vi "Strategy 5_Autotuning PID_With GUI - Copy (2).vi"() -> ()   [LabVIEW 2018]
doc: "This example demonstrates how to use the PID Design function to obtain PID parameters based on measured process."
uses:
  <vilib>/DAQmx/write.llb/DAQmx Write (Digital 1D Bool 1Chan 1Samp).vi
  <vilib>/Instr/_visa.llb/VISA Configure Serial Port (Instr).vi
  <vilib>/DAQmx/create/channels.llb/DAQmx Create Channel (DO-Digital Output).vi
  <vilib>/DAQmx/miscellaneous.llb/DAQmx Fill In Error Info.vi
  <vilib>/addons/control/pid/pid.llb/PID Advanced (DBL).vi
  <vilib>/addons/control/pid/autopid.llb/PID Autotuning Design (Ziegler-Nichols).vi
  <vilib>/addons/control/pid/autopid.llb/PID Autotuning Design (Cohen-Coon).vi
  <vilib>/addons/control/pid/autopid.llb/PID Autotuning Design (Chien-Hrones-Reswick).vi
  <vilib>/addons/control/pid/autopid.llb/PID Autotuning Design (Internal Model Control).vi
  <vilib>/addons/control/pid/NI_PID_autopid.lvlib
  <vilib>/addons/control/pid/NI_PID_pid.lvlib
  <vilib>/ptbypt/NI_PtbyPt.lvlib
panel:
  out "?":bool
  in  "Muscle Control":T1(tab)=enum."M-11"
  out "Tuned PID gains 8":T2={"proportional gain (Kc)"=1.9838195929127882, "integral time (Ti, min)"=0.01995856284686879, "derivative time (Td, min)"=0.0} {"derivative time (Td, min)" format="%#.6g"; "integral time (Ti, min)" format="%#.6g"; "proportional gain (Kc)" format="%#.6g"}
  in  "Accept gain 8":bool
  in  "Control 8":T3(tab)
  in  "Ziegler-Nichols speed 8":u16(ring) items=["Fast", "Normal", "Slow"]
  in  "Tuning specifications 8":u16(ring) items=["Regulator - 0 %", "Regulator -  20%", "Servo - 0%", "Servo - 20%"]
  in  "Multiplicative factor 8":dbl(slide)=1.0 scale=0.01..100.0
  in  "Type of controller 8":u16(ring)=2 items=["P", "PI", "PID"]
  in  "Stop 8":bool
  in  "PID Gains 8":T2={"proportional gain (Kc)"=0.1625, "integral time (Ti, min)"=1.25, "derivative time (Td, min)"=0.0} {"derivative time (Td, min)" format="%#.6g"; "integral time (Ti, min)" format="%#.6g"; "proportional gain (Kc)" format="%#.6g"}
  in  "Autotune 8":bool
  in  "Reinitialize 8":bool
  in  "Excitation 8":dbl=0.5 format="%.2f"
  in  "Automatic 8":bool=TRUE
  in  "MV: 8":dbl(slide)=20.39115328927357 scale=-100.0..100.0
  in  "Set Point 8":dbl(slide) scale=0.0..30.0
  out "PWM Output 8":bool
  out "Real time Data 8":dbl[][](graph)
  in  "Median sample length 17":i32=100
  in  "INLET 2 ON/OFF 2":bool=TRUE
  out "Tuned PID gains 7":T2={"proportional gain (Kc)"=1.9838195929127882, "integral time (Ti, min)"=0.01995856284686879, "derivative time (Td, min)"=0.0} {"derivative time (Td, min)" format="%#.6g"; "integral time (Ti, min)" format="%#.6g"; "proportional gain (Kc)" format="%#.6g"}
  in  "Accept gain 7":bool
  in  "Control 7":T3(tab)
  in  "Ziegler-Nichols speed 7":u16(ring) items=["Fast", "Normal", "Slow"]
  in  "Tuning specifications 7":u16(ring) items=["Regulator - 0 %", "Regulator -  20%", "Servo - 0%", "Servo - 20%"]
  in  "Multiplicative factor 7":dbl(slide)=1.0 scale=0.01..100.0
  in  "Type of controller 7":u16(ring)=2 items=["P", "PI", "PID"]
  in  "Stop 7":bool
  in  "PID Gains 7":T2={"proportional gain (Kc)"=0.1625, "integral time (Ti, min)"=1.25, "derivative time (Td, min)"=0.0} {"derivative time (Td, min)" format="%#.6g"; "integral time (Ti, min)" format="%#.6g"; "proportional gain (Kc)" format="%#.6g"}
  in  "Autotune 7":bool
  in  "Reinitialize 7":bool
  in  "Excitation 7":dbl=0.5 format="%.2f"
  in  "Automatic 7":bool=TRUE
  in  "MV: 7":dbl(slide)=20.39115328927357 scale=-100.0..100.0
  in  "Set Point 7":dbl(slide) scale=0.0..30.0
  out "PWM Output 7":bool
  out "Real time Data 7":dbl[][](graph)
  in  "Median sample length 16":i32=100
  in  "INLET 7 ON/OFF 2":bool=TRUE
  out "Tuned PID gains 6":T2={"proportional gain (Kc)"=1.9838195929127882, "integral time (Ti, min)"=0.01995856284686879, "derivative time (Td, min)"=0.0} {"derivative time (Td, min)" format="%#.6g"; "integral time (Ti, min)" format="%#.6g"; "proportional gain (Kc)" format="%#.6g"}
  in  "Accept gain 6":bool
  in  "Control 6":T3(tab)
  in  "Ziegler-Nichols speed 6":u16(ring) items=["Fast", "Normal", "Slow"]
  in  "Tuning specifications 6":u16(ring) items=["Regulator - 0 %", "Regulator -  20%", "Servo - 0%", "Servo - 20%"]
  in  "Multiplicative factor 6":dbl(slide)=1.0 scale=0.01..100.0
  in  "Type of controller 6":u16(ring)=2 items=["P", "PI", "PID"]
  in  "Stop 6":bool
  in  "PID Gains 6":T2={"proportional gain (Kc)"=0.1625, "integral time (Ti, min)"=1.25, "derivative time (Td, min)"=0.0} {"derivative time (Td, min)" format="%#.6g"; "integral time (Ti, min)" format="%#.6g"; "proportional gain (Kc)" format="%#.6g"}
  in  "Autotune 6":bool
  in  "Reinitialize 6":bool
  in  "Excitation 6":dbl=0.5 format="%.2f"
  in  "Automatic 6":bool=TRUE
  in  "MV: 6":dbl(slide)=20.39115328927357 scale=-100.0..100.0
  in  "Set Point 6":dbl(slide) scale=0.0..30.0
  out "PWM Output 6":bool
  out "Real time Data 6":dbl[][](graph)
  in  "Median sample length 15":i32=100
  in  "INLET 6 ON/OFF 2":bool=TRUE
  out "Tuned PID gains 5":T2={"proportional gain (Kc)"=1.9838195929127882, "integral time (Ti, min)"=0.01995856284686879, "derivative time (Td, min)"=0.0} {"derivative time (Td, min)" format="%#.6g"; "integral time (Ti, min)" format="%#.6g"; "proportional gain (Kc)" format="%#.6g"}
  in  "Accept gain 5":bool
  in  "Control 5":T3(tab)
  in  "Ziegler-Nichols speed 5":u16(ring) items=["Fast", "Normal", "Slow"]
  in  "Tuning specifications 5":u16(ring) items=["Regulator - 0 %", "Regulator -  20%", "Servo - 0%", "Servo - 20%"]
  in  "Multiplicative factor 5":dbl(slide)=1.0 scale=0.01..100.0
  in  "Type of controller 5":u16(ring)=2 items=["P", "PI", "PID"]
  in  "Stop 5":bool
  in  "PID Gains 5":T2={"proportional gain (Kc)"=0.1625, "integral time (Ti, min)"=1.25, "derivative time (Td, min)"=0.0} {"derivative time (Td, min)" format="%#.6g"; "integral time (Ti, min)" format="%#.6g"; "proportional gain (Kc)" format="%#.6g"}
  in  "Autotune 5":bool
  in  "Reinitialize 5":bool
  in  "Excitation 5":dbl=0.5 format="%.2f"
  in  "Automatic 5":bool=TRUE
  in  "MV: 5":dbl(slide)=20.39115328927357 scale=-100.0..100.0
  in  "Set Point 5":dbl(slide) scale=0.0..30.0
  out "PWM Output 5":bool
  out "Real time Data 5":dbl[][](graph)
  in  "Median sample length 14":i32=100
  in  "INLET 8 ON/OFF 2":bool=TRUE
  out "Tuned PID gains 4":T2={"proportional gain (Kc)"=1.9838195929127882, "integral time (Ti, min)"=0.01995856284686879, "derivative time (Td, min)"=0.0} {"derivative time (Td, min)" format="%#.6g"; "integral time (Ti, min)" format="%#.6g"; "proportional gain (Kc)" format="%#.6g"}
  in  "Accept gain 4":bool
  in  "Control 4":T3(tab)
  in  "Ziegler-Nichols speed 4":u16(ring) items=["Fast", "Normal", "Slow"]
  in  "Tuning specifications 4":u16(ring) items=["Regulator - 0 %", "Regulator -  20%", "Servo - 0%", "Servo - 20%"]
  in  "Multiplicative factor 4":dbl(slide)=1.0 scale=0.01..100.0
  in  "Type of controller 4":u16(ring)=2 items=["P", "PI", "PID"]
  in  "Stop 4":bool
  in  "PID Gains 4":T2={"proportional gain (Kc)"=0.1625, "integral time (Ti, min)"=1.25, "derivative time (Td, min)"=0.0} {"derivative time (Td, min)" format="%#.6g"; "integral time (Ti, min)" format="%#.6g"; "proportional gain (Kc)" format="%#.6g"}
  in  "Autotune 4":bool
  in  "Reinitialize 4":bool
  in  "Excitation 4":dbl=0.5 format="%.2f"
  in  "Automatic 4":bool=TRUE
  in  "MV: 4":dbl(slide)=20.39115328927357 scale=-100.0..100.0
  in  "Set Point 4":dbl(slide) scale=0.0..30.0
  out "PWM Output 4":bool
  out "Real time Data 4":dbl[][](graph)
  in  "Median sample length 9":i32=100
  in  "INLET 9 ON/OFF 2":bool=TRUE
  out "Tuned PID gains 3":T2={"proportional gain (Kc)"=1.9838195929127882, "integral time (Ti, min)"=0.01995856284686879, "derivative time (Td, min)"=0.0} {"derivative time (Td, min)" format="%#.6g"; "integral time (Ti, min)" format="%#.6g"; "proportional gain (Kc)" format="%#.6g"}
  in  "Accept gain 3":bool
  in  "Control 3":T3(tab)
  in  "Ziegler-Nichols speed 3":u16(ring) items=["Fast", "Normal", "Slow"]
  in  "Tuning specifications 3":u16(ring) items=["Regulator - 0 %", "Regulator -  20%", "Servo - 0%", "Servo - 20%"]
  in  "Multiplicative factor 3":dbl(slide)=1.0 scale=0.01..100.0
  in  "Type of controller 3":u16(ring)=2 items=["P", "PI", "PID"]
  in  "Stop 3":bool
  in  "PID Gains 3":T2={"proportional gain (Kc)"=0.1625, "integral time (Ti, min)"=1.25, "derivative time (Td, min)"=0.0} {"derivative time (Td, min)" format="%#.6g"; "integral time (Ti, min)" format="%#.6g"; "proportional gain (Kc)" format="%#.6g"}
  in  "Autotune 3":bool
  in  "Reinitialize 3":bool
  in  "Excitation 3":dbl=0.5 format="%.2f"
  in  "Automatic 3":bool=TRUE
  in  "MV: 3":dbl(slide)=20.39115328927357 scale=-100.0..100.0
  in  "Set Point 3":dbl(slide) scale=0.0..30.0
  out "PWM Output 3":bool
  out "Real time Data 3":dbl[][](graph)
  in  "Median sample length 13":i32=100
  in  "INLET 10 ON/OFF":bool=TRUE
  in  "INLET":bool=TRUE
  out "PWM Output":bool
  out "Real time Data":dbl[][](graph)
  in  "MV:":dbl(slide)=20.39115328927357 scale=-100.0..100.0
  in  "Set Point":dbl(slide) scale=0.0..30.0
  in  "Median sample length":i32=100
  in  "Excitation":dbl=0.5 format="%.2f"
  in  "Type of controller":u16(ring)=2 items=["P", "PI", "PID"]
  in  "Control":T3(tab)
  in  "Ziegler-Nichols speed":u16(ring) items=["Fast", "Normal", "Slow"]
  in  "Tuning specifications":u16(ring) items=["Regulator - 0 %", "Regulator -  20%", "Servo - 0%", "Servo - 20%"]
  in  "Multiplicative factor":dbl(slide)=1.0 scale=0.01..100.0
  in  "Automatic":bool=TRUE
  in  "Reinitialize":bool
  in  "Accept gain":bool
  out "Tuned PID gains":T2={"proportional gain (Kc)"=1.9838195929127882, "integral time (Ti, min)"=0.01995856284686879, "derivative time (Td, min)"=0.0} {"derivative time (Td, min)" format="%#.6g"; "integral time (Ti, min)" format="%#.6g"; "proportional gain (Kc)" format="%#.6g"}
  in  "Autotune":bool
  in  "PID Gains":T2={"proportional gain (Kc)"=0.1625, "integral time (Ti, min)"=1.25, "derivative time (Td, min)"=0.0} {"derivative time (Td, min)" format="%#.6g"; "integral time (Ti, min)" format="%#.6g"; "proportional gain (Kc)" format="%#.6g"}
  in  "Stop":bool
  out "Tuned PID gains 2":T2={"proportional gain (Kc)"=1.9838195929127882, "integral time (Ti, min)"=0.01995856284686879, "derivative time (Td, min)"=0.0} {"derivative time (Td, min)" format="%#.6g"; "integral time (Ti, min)" format="%#.6g"; "proportional gain (Kc)" format="%#.6g"}
  in  "Accept gain 2":bool
  in  "Control 2":T3(tab)
  in  "Ziegler-Nichols speed 2":u16(ring) items=["Fast", "Normal", "Slow"]
  in  "Tuning specifications 2":u16(ring) items=["Regulator - 0 %", "Regulator -  20%", "Servo - 0%", "Servo - 20%"]
  in  "Multiplicative factor 2":dbl(slide)=1.0 scale=0.01..100.0
  in  "Type of controller 2":u16(ring)=2 items=["P", "PI", "PID"]
  in  "Stop 2":bool
  in  "PID Gains 2":T2={"proportional gain (Kc)"=0.1625, "integral time (Ti, min)"=1.25, "derivative time (Td, min)"=0.0} {"derivative time (Td, min)" format="%#.6g"; "integral time (Ti, min)" format="%#.6g"; "proportional gain (Kc)" format="%#.6g"}
  in  "Autotune 2":bool
  in  "Reinitialize 2":bool
  in  "Excitation 2":dbl=0.5 format="%.2f"
  in  "Automatic 2":bool=TRUE
  in  "MV: 2":dbl(slide)=20.39115328927357 scale=-100.0..100.0
  in  "Set Point 2":dbl(slide) scale=0.0..30.0
  out "PWM Output 2":bool
  out "Real time Data 2":dbl[][](graph)
  in  "Median sample length 12":i32=100
  in  "INLET 12 ON/OFF":bool=TRUE
  in  "M-11":i32=5
  in  "M-12":i32=5
  in  "M-10":i32=5
  in  "M-9":i32=5
  in  "M-8":i32=5
  in  "M-6":i32=5
  in  "M-7":i32=5
  in  "M-2":i32=5
  out "Identified Plant Parameters":T4={"Plant Gain (K)"=1.7609511324977591, "Time Constant (T)"=1.9621978490901302, "Dead Time (L)"=0.22467425343567116}
  out "Control Output":dbl[](graph)
  out "Measurement":dbl[](graph)
  out "Stimulus operating point":dbl=20.314221540357543
  out "Response operating point":dbl=51.08345461694337
  out "Stimulus operating point 2":dbl=20.314221540357543
  out "Response operating point 2":dbl=51.08345461694337
  out "Identified Plant Parameters 2":T4={"Plant Gain (K)"=1.7609511324977591, "Time Constant (T)"=1.9621978490901302, "Dead Time (L)"=0.22467425343567116}
  out "Control Output 2":dbl[](graph)
  out "Measurement 2":dbl[](graph)
  out "Stimulus operating point 3":dbl=20.314221540357543
  out "Response operating point 3":dbl=51.08345461694337
  out "Identified Plant Parameters 3":T4={"Plant Gain (K)"=1.7609511324977591, "Time Constant (T)"=1.9621978490901302, "Dead Time (L)"=0.22467425343567116}
  out "Control Output 3":dbl[](graph)
  out "Measurement 3":dbl[](graph)
  out "Stimulus operating point 4":dbl=20.314221540357543
  out "Response operating point 4":dbl=51.08345461694337
  out "Identified Plant Parameters 4":T4={"Plant Gain (K)"=1.7609511324977591, "Time Constant (T)"=1.9621978490901302, "Dead Time (L)"=0.22467425343567116}
  out "Control Output 4":dbl[](graph)
  out "Measurement 4":dbl[](graph)
  out "Stimulus operating point 5":dbl=20.314221540357543
  out "Response operating point 5":dbl=51.08345461694337
  out "Identified Plant Parameters 5":T4={"Plant Gain (K)"=1.7609511324977591, "Time Constant (T)"=1.9621978490901302, "Dead Time (L)"=0.22467425343567116}
  out "Control Output 5":dbl[](graph)
  out "Measurement 5":dbl[](graph)
  out "Stimulus operating point 6":dbl=20.314221540357543
  out "Response operating point 6":dbl=51.08345461694337
  out "Identified Plant Parameters 6":T4={"Plant Gain (K)"=1.7609511324977591, "Time Constant (T)"=1.9621978490901302, "Dead Time (L)"=0.22467425343567116}
  out "Control Output 6":dbl[](graph)
  out "Measurement 6":dbl[](graph)
  out "Stimulus operating point 7":dbl=20.314221540357543
  out "Response operating point 7":dbl=51.08345461694337
  out "Identified Plant Parameters 7":T4={"Plant Gain (K)"=1.7609511324977591, "Time Constant (T)"=1.9621978490901302, "Dead Time (L)"=0.22467425343567116}
  out "Control Output 7":dbl[](graph)
  out "Measurement 7":dbl[](graph)
  out "Stimulus operating point 8":dbl=20.314221540357543
  out "Response operating point 8":dbl=51.08345461694337
  out "Identified Plant Parameters 8":T4={"Plant Gain (K)"=1.7609511324977591, "Time Constant (T)"=1.9621978490901302, "Dead Time (L)"=0.22467425343567116}
  out "Control Output 8":dbl[](graph)
  out "Measurement 8":dbl[](graph)
  in  "XYZAER":T5(array[cluster]) {"r" format="%1_6f"; "e" format="%1_6f"; "a" format="%1_6f"; "z" format="%1_6f"; "y" format="%1_6f"; "x" format="%1_6f"}
  out "Connected":bool
  out "Start Time Text":string
  out "Stop Time Text":string
  out "Elapsed Time Text":string
  out "HostFrameCount":u32
  out "Running":bool
  out "Loop Iter":i32
  out "PnoData":bool
  in  "stop":bool
  out "error out":errorcluster {"code" format="%.0x"}
  out "Position Sensor Data":cluster{dbl, "x":sgl}[](graph)
  out "Sensor Raw Value 2":i32
  in  "COM Port-Sensor 2":refnum<visa-resource-name>="COM5"
  in  "upper/lower infle":enum32{"Page 1", "Page 2"}(tab)
  out "Force in Kilograms":dbl(graph)
  out "Force in Newtons":dbl(graph)
  in  "lower/upper infle":enum32{"Page 1", "Page 2"}(tab)
  out "Force in Newtons 2":dbl(graph)
  out "Force in Kilograms 2":dbl(graph)
  in  "COM Port-Sensor 1":refnum<visa-resource-name>="COM4"
  out "Sensor Raw Value":i32
  in  "Tab Control":T6(tab)
  in  "Instructions":string="Overview: This example demonstrates how to use the PID Autotuning Design to obtain PID parameters based on setpoint and process variable collected in another loop.\nInstructions:\n1. Run the VI and wait until the process variable (PV) reaches near setpoint (SP).\n2.  In the PID Autotuning Design section, select the type of algorithm, type of controller and excitation amplitude for the 'open loop step response'. Then, click Autotune to start the process. Select the Identified Plant Parameter tab and see the results from the identification.\n3.  When the tuned PID gains do not change anymore, the identification is done and you have the option to accept by clicking Accept gain, which will transfer the new gain to PID Gains.\n4. Click the Autotune button again to go back to the automatic control state. You can try different options and repeat this process.\n5. Click Stop to stop the VI.\n"
  in  "Instructions 2":string="Overview: This example demonstrates how to use the PID Autotuning Design to obtain PID parameters based on setpoint and process variable collected in another loop.\nInstructions:\n1. Run the VI and wait until the process variable (PV) reaches near setpoint (SP).\n2.  In the PID Autotuning Design section, select the type of algorithm, type of controller and excitation amplitude for the 'open loop step response'. Then, click Autotune to start the process. Select the Identified Plant Parameter tab and see the results from the identification.\n3.  When the tuned PID gains do not change anymore, the identification is done and you have the option to accept by clicking Accept gain, which will transfer the new gain to PID Gains.\n4. Click the Autotune button again to go back to the automatic control state. You can try different options and repeat this process.\n5. Click Stop to stop the VI.\n"
  in  "Instructions 3":string="Overview: This example demonstrates how to use the PID Autotuning Design to obtain PID parameters based on setpoint and process variable collected in another loop.\nInstructions:\n1. Run the VI and wait until the process variable (PV) reaches near setpoint (SP).\n2.  In the PID Autotuning Design section, select the type of algorithm, type of controller and excitation amplitude for the 'open loop step response'. Then, click Autotune to start the process. Select the Identified Plant Parameter tab and see the results from the identification.\n3.  When the tuned PID gains do not change anymore, the identification is done and you have the option to accept by clicking Accept gain, which will transfer the new gain to PID Gains.\n4. Click the Autotune button again to go back to the automatic control state. You can try different options and repeat this process.\n5. Click Stop to stop the VI.\n"
  # "Pressure Alarm"
  # "Position Sensor Data"
  # "Force Sensor Data"
  # "PID Controller"
  # "PID Autotuning Design"
  # "No additional parameters"
  # "PID Controller"
  # "PID Autotuning Design"
  # "No additional parameters"
  # "PID Controller"
  # "PID Autotuning Design"
  # "No additional parameters"
  # "Muscle Control"
  # "PID Controller"
  # "PID Autotuning Design"
  # "No additional parameters"
  # "PID Controller"
  # "PID Autotuning Design"
  # "No additional parameters"
  # "PID Controller"
  # "PID Autotuning Design"
  # "No additional parameters"
  # "Muscle Control"
  # "PID Controller"
  # "PID Autotuning Design"
  # "No additional parameters"
  # "PID Controller"
  # "PID Autotuning Design"
  # "No additional parameters"
  # "Pressure Cut Off to trigger the alarm"
  # "M-11"
  # "M-12"
  # "M-10"
  # "M-9"
  # "M-8"
  # "M-6"
  # "M-7"
  # "M-2"
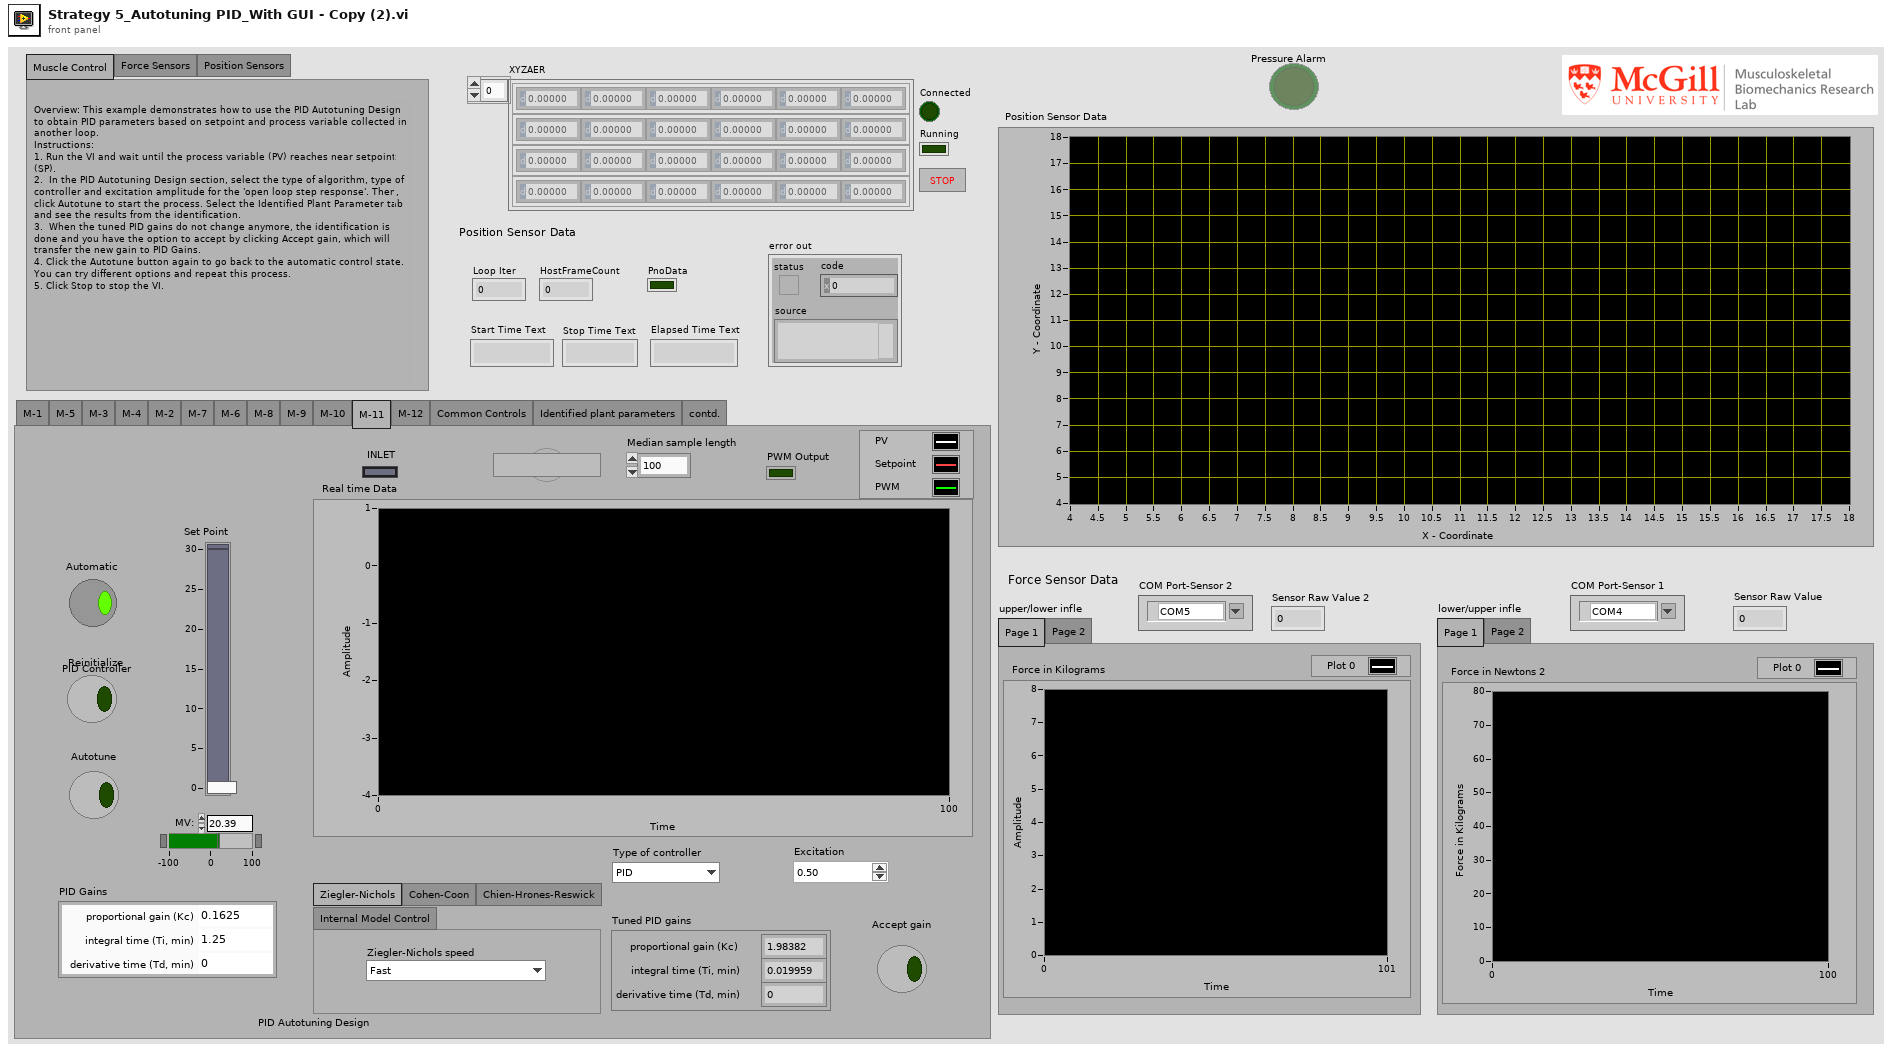
[diagram p1: front panel]
types:
  T1 = enum32{"M-1", "M-5", "M-3", "M-4", "M-2", "M-7", "M-6", "M-8", "M-9", "M-10", "M-11", "M-12", "Common Controls", "Identified plant parameters", "contd."}
  T2 = cluster{"proportional gain (Kc)":dbl, "integral time (Ti, min)":dbl, "derivative time (Td, min)":dbl}
  T3 = enum32{"Ziegler-Nichols", "Cohen-Coon", "Chien-Hrones-Reswick", "Internal Model Control"}
  T4 = cluster{"Plant Gain (K)":dbl, "Time Constant (T)":dbl, "Dead Time (L)":dbl}
  T5 = cluster{"x":sgl, "y":sgl, "z":sgl, "a":sgl, "e":sgl, "r":sgl}[]
  T6 = enum32{"Muscle Control", "Force Sensors", "Position Sensors"}
  T7 = cluster{"static gain":dbl, "lag (s)":dbl, "deadtime (s)":dbl, "load":dbl, "deadband":dbl, "sensor noise":dbl, "initial PV":dbl, "plant noise":dbl}
  T8 = cluster{"x":sgl, "y":sgl, "z":sgl, "a":sgl, "e":sgl, "r":sgl}
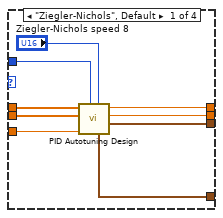
[diagram p2: hidden frame]
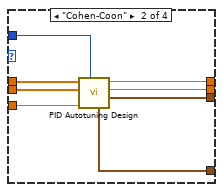
[diagram p3: hidden frame]
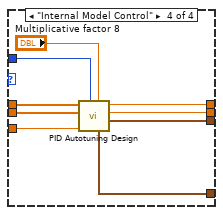
[diagram p4: hidden frame]
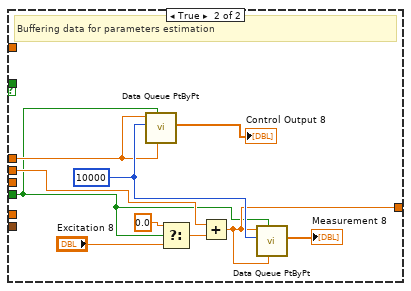
[diagram p6: hidden frame]
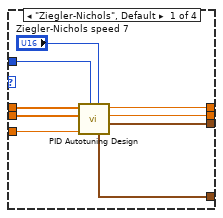
[diagram p7: hidden frame]
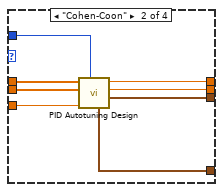
[diagram p8: hidden frame]
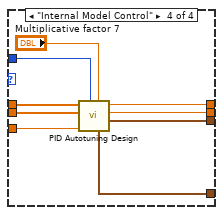
[diagram p9: hidden frame]
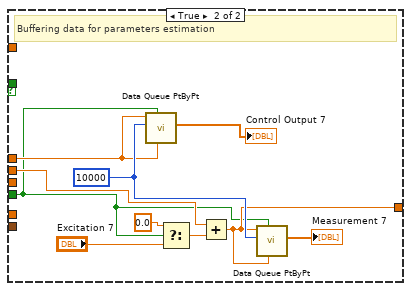
[diagram p11: hidden frame]
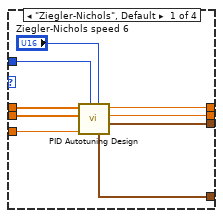
[diagram p12: hidden frame]
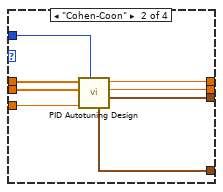
[diagram p13: hidden frame]
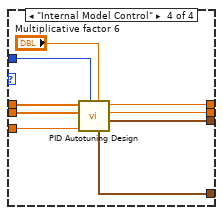
[diagram p14: hidden frame]
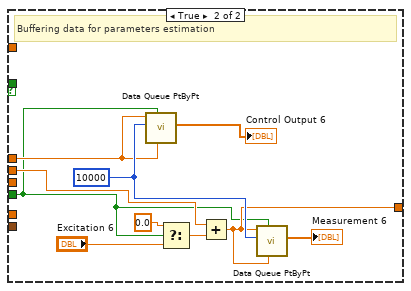
[diagram p16: hidden frame]
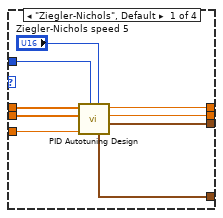
[diagram p17: hidden frame]
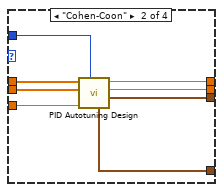
[diagram p18: hidden frame]
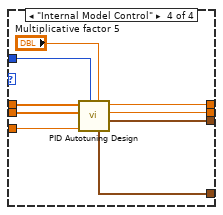
[diagram p19: hidden frame]
diagram:
  w3 = 0.0 ("output")
  w6 = FALSE ("Stop")
  w9 = 0.0 ("output")
  w12 = FALSE ("Stop")
  w15 = 0.0 ("output")
  w18 = FALSE ("Stop")
  w21 = 0.0 ("output")
  w24 = FALSE ("Stop")
  w27 = 0.0 ("output")
  w30 = FALSE ("Stop")
  w33 = 0.0 ("output")
  w36 = FALSE ("Stop")
  w39 = 0.0 ("output")
  w42 = FALSE ("Stop")
  w50 = 2400  # BufferFrameCount
  w84 = 0.0 ("output")
  w87 = FALSE ("Stop")
  # "Muscle-2 PID CONTROL LOOP (Auto Tuning)"
  # "Muscle-7 PID CONTROL LOOP (Auto Tuning)"
  # "Muscle-6 PID CONTROL LOOP (Auto Tuning)"
  # "Muscle-8 PID CONTROL LOOP (Auto Tuning)"
  # "Muscle-9 PID CONTROL LOOP (Auto Tuning)"
  # "Muscle-10 PID CONTROL LOOP (Auto Tuning)"
  # "Muscle-12 PID CONTROL LOOP (Auto Tuning)"
  # "Muscle-11 PID CONTROL LOOP (Auto Tuning)"
  # "FORCE SENSOR CONTROL LOOP"
  # "POSITION SENSOR CONTROL LOOP"
  # "Pressure Alarm"
  # "8. Close Tracker connection."
  # "3. Query Max num sensors supported by the tracker."
  # "4. Allocate raw buffer to hold 2400 frames of data."
  # "5. Start Continuous mode."
  # "7. Stop Continuous mode."
  # "6. Start the loop. Loop exits when Stop Button is hit."
  n1 = call "DAQ Assistant"() -> ("data"=w1:dynamicdata)  [unwired: 17 in, 2 out]
  n2 = while {
    shift-left: 0.0 ("Plant Output") -> [w153]
    shift-right: [w148] -> _
    tunnel: w18 -> [_]
    shift-right: [w134] -> _
    shift-left: 0.01 -> [w132]
    shift-right: [w106] -> _
    shift-left: TRUE -> [w131]
    shift-right: [w108] -> _
    shift-left: w15 -> [w130]
    shift-right: [w133] -> _
    shift-left: w15 -> [w129]
    tunnel: [w103] -> w14
    tunnel: w1 -> [w89]
    stop <- "Stop 6" stop-if-true
    w94 = 1 items=["one channel for each line", "one channel for all lines"] ("line grouping")
    w103 = 0.05 ("Sampling Time dt (s)")
    w112 = 1 items=["one channel for each line", "one channel for all lines"] ("line grouping")
    w120 = 0.5 ("x")
    w147 = T7 {"static gain"=2.5, "lag (s)"=2.5, "deadtime (s)"=0.01, "load"=0.0, "deadband"=0.0, "sensor noise"=0.0, "initial PV"=30.0, "plant noise"=0.0}  # Process parameters
    w149 = FALSE  # Integrator ?
    # "C."
    # "Inlet 11"
    # "Exhaust 6"
    # "B."
    # "A."
    # "A.Output to PWM Logic \nB. Simulated Plant\nC. Draw Chart"
    # "Main PID Loop Control"
    n3 = Multiply(x=w103, y=1000.0) -> (x*y=w146:dbl)
    n4 = Not(x="Autotune 6") -> (.not. x?=w150:bool)
    n5 = feedback #1() -> (w155:bool)  [unwired: 1 in]
    n6 = feedback-in #1("Autotune 6") -> ()
    n7 = Wait Until Next ms Multiple(millisecond multiple=w146) -> ()  [unwired: 1 out]
    n8 = Exclusive Or(1:w155, 2:"Autotune 6") -> (0:w154:bool)
    n9 = feedback #2() -> (w152:dbl)  [unwired: 1 in]
    n10 = Multiply(x=w89, y=-1000.0) -> (x*y=w136:dynamicdata)
    n11 = call <vilib>:"Median PtByPt.vi"("sample length"="Median sample length 15", "x"=w136) -> ("median"=w135:dbl)  [unwired: 2 in, 1 out]
    n12 = Square(x=w135) -> (x^2=w143:dbl)
    n13 = Multiply(x=w135, y=-39.646) -> (x*y=w139:dbl)
    n14 = Multiply(x=w143, y=0.2324) -> (x*y=w140:dbl)
    n15 = Add(x=w139, y=w140) -> (x+y=w138:dbl)
    n16 = Add(x=1678.0, y=w138) -> (x+y=w101:dbl)
    n17 = case shown="False" "Autotune 6" {
      tunnel: w103 -> [w170 _]
      tunnel: [w159 w175] -> w108
      tunnel: w153 -> [_ w174]
      tunnel: "PID Gains 6" -> [w169 _]
      tunnel: "Reinitialize 6" -> [w166 _]
      tunnel: w154 -> [w168 w173]
      tunnel: w152 -> [_ w177]
      tunnel: w101 -> [w162 _]
      tunnel: "Set Point 6" -> [w161 _]
      frame False {
        # "This code is to have 'bumpless' transfer from autotuning"
        n18 = Not(x=w168) -> (.not. x?=w165:bool)
        n19 = And(x="Automatic 6", y=w165) -> (x .and. y?=w167:bool)
        n20 = call-poly <vilib>:"PID Advanced.vi"("setpoint"=w161, "auto? (T)"=w167, "manual control"="MV: 6", "process variable"=w162, "alpha"=10.0, "PID gains"=w169, "dt (s)"=w170, "reinitialize? (F)"=w166) -> ("output"=w159:dbl)  [unwired: 6 in, 1 out]
      }
      frame True {
        w180 = 10000 ("sample length")
        # "Buffering data for parameters estimation"
        n21 = call <vilib>:"Data Queue PtByPt.vi"("initial queue element"=w174, "initialize"=w173, "sample length"=w180, "input data point"=w174) -> ("Current Queue"=→"Control Output 6":dbl[])  [unwired: 3 in, 4 out]
        n22 = Select(t=0.0, s=w173, f="Excitation 6") -> (s? t:f=w178:dbl)
        n23 = Add(x=w177, y=w178) -> (x+y=w175:dbl)
        n24 = call <vilib>:"Data Queue PtByPt.vi"("initial queue element"=w175, "initialize"=w173, "sample length"=w180, "input data point"=w175) -> ("Current Queue"=→"Measurement 6":dbl[])  [unwired: 3 in, 4 out]
      }
    }
    n25 = feedback-in #2(w108, w150) -> ()
    n26 = Greater?(x=w101, y="M-6") -> ()  [unwired: 1 out]
    n27 = Add(x=w132, y=w120) -> (x+y=w121:dbl)
    n28 = Subtract(x=w132, y=w120) -> (x-y=w119:dbl)
    n29 = Equal?(x=w130, y=w108) -> (x = y?=w127:bool)
    n30 = Greater?(x=w108, y=w130) -> (0:w126:bool)
    n31 = Select(t=w131, s=w127, f=w126) -> (s? t:f=w106:bool)
    "PWM Output 6" <- w106
    n32 = call "Plant System.vi"("Integrator ?"=w149, "Plant Input"=w108, "dt (s)"=w103, "process parameters"=w147) -> ("Plant Output"=w148:dbl)  [unwired: 11 in]
    n33 = Increment(x="Set Point 6") -> (x+1=w125:dbl)
    n34 = Decrement(x="Set Point 6") -> (x-1=w124:dbl)
    n35 = Select(t=w121, s=w106, f=w119) -> (s? t:f=w134:dbl)
    n36 = Select(t=w125, s=w106, f=w124) -> (s? t:f=w123:dbl)
    n37 = Not(x=w106) -> (.not. x?=w105:bool)
    n38 = call-poly <vilib>:"DAQmx Create Virtual Channel.vi"("lines"=tag "cDAQ1Mod1/port0/line4", "line grouping"=w112) -> ("task out"=w114:refnum<k21>, "error out"=w113:errorcluster)  [unwired: 12 in]
    n39 = call-poly <vilib>:"DAQmx Create Virtual Channel.vi"("lines"=tag "cDAQ1Mod2/port0/line4", "line grouping"=w94) -> ("task out"=w96:refnum<k21>, "error out"=w95:errorcluster)  [unwired: 12 in]
    n40 = Build Array(w101, "Set Point 6", w123) -> (w122:dbl[])
    n41 = Initialize Array("INLET 6 ON/OFF 2", 1 ("dimension size")) -> (w91:bool[])
    n42 = Initialize Array(w105, 1 ("dimension size")) -> (w109:bool[])
    n43 = local write "MV: 6"(w108) -> ()
    n44 = Add(x=w129, y=w132) -> (x+y=w133:dbl)
    n45 = Build Array(w122) -> (→"Real time Data 6":dbl[][])
    n46 = call-poly <vilib>:"DAQmx Write.vi"("task/channels in"=w114, "auto start"=TRUE, "data"=w109, "error in"=w113) -> ("task out"=w116:refnum<k21>, "error out"=w117:errorcluster)  [unwired: 9 in, 1 out]
    n47 = call-poly <vilib>:"DAQmx Write.vi"("task/channels in"=w96, "auto start"=TRUE, "data"=w91, "error in"=w95) -> ("task out"=w98:refnum<k21>, "error out"=w99:errorcluster)  [unwired: 9 in, 1 out]
    n48 = call <vilib>:"DAQmx Clear Task.vi"("task in"=w116, "error in"=w117) -> ("error out"=w111:errorcluster)  [unwired: 13 in]
    n49 = call <vilib>:"DAQmx Clear Task.vi"("task in"=w98, "error in"=w99) -> ("error out"=w93:errorcluster)  [unwired: 13 in]
    n50 = call <vilib>:"Simple Error Handler.vi"("error in (no error)"=w111) -> ()  [unwired: 4 in, 5 out]
    n51 = call <vilib>:"Simple Error Handler.vi"("error in (no error)"=w93) -> ()  [unwired: 4 in, 5 out]
  }
  n52 = while {
    shift-left: 0.0 ("Plant Output") -> [w245]
    shift-right: [w240] -> _
    tunnel: w30 -> [_]
    shift-right: [w226] -> _
    shift-left: 0.01 -> [w224]
    shift-right: [w198] -> _
    shift-left: TRUE -> [w223]
    shift-right: [w200] -> _
    shift-left: w27 -> [w222]
    shift-right: [w225] -> _
    shift-left: w27 -> [w221]
    tunnel: [w195] -> w26
    tunnel: w1 -> [w181]
    stop <- "Stop 4" stop-if-true
    w186 = 1 items=["one channel for each line", "one channel for all lines"] ("line grouping")
    w195 = 0.05 ("Sampling Time dt (s)")
    w204 = 1 items=["one channel for each line", "one channel for all lines"] ("line grouping")
    w212 = 0.5 ("x")
    w239 = T7 {"static gain"=2.5, "lag (s)"=2.5, "deadtime (s)"=0.01, "load"=0.0, "deadband"=0.0, "sensor noise"=0.0, "initial PV"=30.0, "plant noise"=0.0}  # Process parameters
    w241 = FALSE  # Integrator ?
    # "C."
    # "Inlet 11"
    # "Exhaust 9"
    # "B."
    # "A."
    # "A.Output to PWM Logic \nB. Simulated Plant\nC. Draw Chart"
    # "Main PID Loop Control"
    n53 = Multiply(x=w195, y=1000.0) -> (x*y=w238:dbl)
    n54 = Not(x="Autotune 4") -> (.not. x?=w242:bool)
    n55 = feedback #3() -> (w247:bool)  [unwired: 1 in]
    n56 = feedback-in #3("Autotune 4") -> ()
    n57 = Wait Until Next ms Multiple(millisecond multiple=w238) -> ()  [unwired: 1 out]
    n58 = Exclusive Or(1:w247, 2:"Autotune 4") -> (0:w246:bool)
    n59 = feedback #4() -> (w244:dbl)  [unwired: 1 in]
    n60 = Multiply(x=w181, y=-1000.0) -> (x*y=w228:dynamicdata)
    n61 = call <vilib>:"Median PtByPt.vi"("sample length"="Median sample length 9", "x"=w228) -> ("median"=w227:dbl)  [unwired: 2 in, 1 out]
    n62 = Square(x=w227) -> (x^2=w235:dbl)
    n63 = Multiply(x=w227, y=-39.646) -> (x*y=w231:dbl)
    n64 = Multiply(x=w235, y=0.2324) -> (x*y=w232:dbl)
    n65 = Add(x=w231, y=w232) -> (x+y=w230:dbl)
    n66 = Add(x=1678.0, y=w230) -> (x+y=w193:dbl)
    n67 = case shown="False" "Autotune 4" {
      tunnel: w195 -> [w262 _]
      tunnel: [w251 w267] -> w200
      tunnel: w245 -> [_ w266]
      tunnel: "PID Gains 4" -> [w261 _]
      tunnel: "Reinitialize 4" -> [w258 _]
      tunnel: w246 -> [w260 w265]
      tunnel: w244 -> [_ w269]
      tunnel: w193 -> [w254 _]
      tunnel: "Set Point 4" -> [w253 _]
      frame False {
        # "This code is to have 'bumpless' transfer from autotuning"
        n68 = Not(x=w260) -> (.not. x?=w257:bool)
        n69 = And(x="Automatic 4", y=w257) -> (x .and. y?=w259:bool)
        n70 = call-poly <vilib>:"PID Advanced.vi"("setpoint"=w253, "auto? (T)"=w259, "manual control"="MV: 4", "process variable"=w254, "alpha"=10.0, "PID gains"=w261, "dt (s)"=w262, "reinitialize? (F)"=w258) -> ("output"=w251:dbl)  [unwired: 6 in, 1 out]
      }
      frame True {
        w272 = 10000 ("sample length")
        # "Buffering data for parameters estimation"
        n71 = call <vilib>:"Data Queue PtByPt.vi"("initial queue element"=w266, "initialize"=w265, "sample length"=w272, "input data point"=w266) -> ("Current Queue"=→"Control Output 4":dbl[])  [unwired: 3 in, 4 out]
        n72 = Select(t=0.0, s=w265, f="Excitation 4") -> (s? t:f=w270:dbl)
        n73 = Add(x=w269, y=w270) -> (x+y=w267:dbl)
        n74 = call <vilib>:"Data Queue PtByPt.vi"("initial queue element"=w267, "initialize"=w265, "sample length"=w272, "input data point"=w267) -> ("Current Queue"=→"Measurement 4":dbl[])  [unwired: 3 in, 4 out]
      }
    }
    n75 = feedback-in #4(w200, w242) -> ()
    n76 = Greater?(x=w193, y="M-9") -> ()  [unwired: 1 out]
    n77 = Add(x=w224, y=w212) -> (x+y=w213:dbl)
    n78 = Subtract(x=w224, y=w212) -> (x-y=w211:dbl)
    n79 = Equal?(x=w222, y=w200) -> (x = y?=w219:bool)
    n80 = Greater?(x=w200, y=w222) -> (0:w218:bool)
    n81 = Select(t=w223, s=w219, f=w218) -> (s? t:f=w198:bool)
    "PWM Output 4" <- w198
    n82 = call "Plant System.vi"("Integrator ?"=w241, "Plant Input"=w200, "dt (s)"=w195, "process parameters"=w239) -> ("Plant Output"=w240:dbl)  [unwired: 11 in]
    n83 = Increment(x="Set Point 4") -> (x+1=w217:dbl)
    n84 = Decrement(x="Set Point 4") -> (x-1=w216:dbl)
    n85 = Select(t=w213, s=w198, f=w211) -> (s? t:f=w226:dbl)
    n86 = Select(t=w217, s=w198, f=w216) -> (s? t:f=w215:dbl)
    n87 = Not(x=w198) -> (.not. x?=w197:bool)
    n88 = call-poly <vilib>:"DAQmx Create Virtual Channel.vi"("lines"=tag "cDAQ1Mod1/port0/line3", "line grouping"=w204) -> ("task out"=w206:refnum<k21>, "error out"=w205:errorcluster)  [unwired: 12 in]
    n89 = call-poly <vilib>:"DAQmx Create Virtual Channel.vi"("lines"=tag "cDAQ1Mod2/port0/line3", "line grouping"=w186) -> ("task out"=w188:refnum<k21>, "error out"=w187:errorcluster)  [unwired: 12 in]
    n90 = Build Array(w193, "Set Point 4", w215) -> (w214:dbl[])
    n91 = Initialize Array("INLET 9 ON/OFF 2", 1 ("dimension size")) -> (w183:bool[])
    n92 = Initialize Array(w197, 1 ("dimension size")) -> (w201:bool[])
    n93 = local write "MV: 4"(w200) -> ()
    n94 = Add(x=w221, y=w224) -> (x+y=w225:dbl)
    n95 = Build Array(w214) -> (→"Real time Data 4":dbl[][])
    n96 = call-poly <vilib>:"DAQmx Write.vi"("task/channels in"=w206, "auto start"=TRUE, "data"=w201, "error in"=w205) -> ("task out"=w208:refnum<k21>, "error out"=w209:errorcluster)  [unwired: 9 in, 1 out]
    n97 = call-poly <vilib>:"DAQmx Write.vi"("task/channels in"=w188, "auto start"=TRUE, "data"=w183, "error in"=w187) -> ("task out"=w190:refnum<k21>, "error out"=w191:errorcluster)  [unwired: 9 in, 1 out]
    n98 = call <vilib>:"DAQmx Clear Task.vi"("task in"=w208, "error in"=w209) -> ("error out"=w203:errorcluster)  [unwired: 13 in]
    n99 = call <vilib>:"DAQmx Clear Task.vi"("task in"=w190, "error in"=w191) -> ("error out"=w185:errorcluster)  [unwired: 13 in]
    n100 = call <vilib>:"Simple Error Handler.vi"("error in (no error)"=w203) -> ()  [unwired: 4 in, 5 out]
    n101 = call <vilib>:"Simple Error Handler.vi"("error in (no error)"=w185) -> ()  [unwired: 4 in, 5 out]
  }
  n102 = while {
    shift-left: 0.0 ("Plant Output") -> [w337]
    shift-right: [w332] -> _
    tunnel: w36 -> [_]
    shift-right: [w318] -> _
    shift-left: 0.01 -> [w316]
    shift-right: [w290] -> _
    shift-left: TRUE -> [w315]
    shift-right: [w292] -> _
    shift-left: w33 -> [w314]
    shift-right: [w317] -> _
    shift-left: w33 -> [w313]
    tunnel: [w287] -> w32
    tunnel: w1 -> [w273]
    stop <- "Stop 3" stop-if-true
    w278 = 1 items=["one channel for each line", "one channel for all lines"] ("line grouping")
    w287 = 0.05 ("Sampling Time dt (s)")
    w296 = 1 items=["one channel for each line", "one channel for all lines"] ("line grouping")
    w304 = 0.5 ("x")
    w331 = T7 {"static gain"=2.5, "lag (s)"=2.5, "deadtime (s)"=0.01, "load"=0.0, "deadband"=0.0, "sensor noise"=0.0, "initial PV"=30.0, "plant noise"=0.0}  # Process parameters
    w333 = FALSE  # Integrator ?
    # "C."
    # "Inlet 11"
    # "Exhaust 10"
    # "B."
    # "A."
    # "A.Output to PWM Logic \nB. Simulated Plant\nC. Draw Chart"
    # "Main PID Loop Control"
    n103 = Multiply(x=w287, y=1000.0) -> (x*y=w330:dbl)
    n104 = Not(x="Autotune 3") -> (.not. x?=w334:bool)
    n105 = feedback #5() -> (w339:bool)  [unwired: 1 in]
    n106 = feedback-in #5("Autotune 3") -> ()
    n107 = Wait Until Next ms Multiple(millisecond multiple=w330) -> ()  [unwired: 1 out]
    n108 = Exclusive Or(1:w339, 2:"Autotune 3") -> (0:w338:bool)
    n109 = feedback #6() -> (w336:dbl)  [unwired: 1 in]
    n110 = Multiply(x=w273, y=-1000.0) -> (x*y=w320:dynamicdata)
    n111 = call <vilib>:"Median PtByPt.vi"("sample length"="Median sample length 13", "x"=w320) -> ("median"=w319:dbl)  [unwired: 2 in, 1 out]
    n112 = Square(x=w319) -> (x^2=w327:dbl)
    n113 = Multiply(x=w319, y=-39.646) -> (x*y=w323:dbl)
    n114 = Multiply(x=w327, y=0.2324) -> (x*y=w324:dbl)
    n115 = Add(x=w323, y=w324) -> (x+y=w322:dbl)
    n116 = Add(x=1678.0, y=w322) -> (x+y=w285:dbl)
    n117 = case shown="False" "Autotune 3" {
      tunnel: w287 -> [w354 _]
      tunnel: [w343 w359] -> w292
      tunnel: w337 -> [_ w358]
      tunnel: "PID Gains 3" -> [w353 _]
      tunnel: "Reinitialize 3" -> [w350 _]
      tunnel: w338 -> [w352 w357]
      tunnel: w336 -> [_ w361]
      tunnel: w285 -> [w346 _]
      tunnel: "Set Point 3" -> [w345 _]
      frame False {
        # "This code is to have 'bumpless' transfer from autotuning"
        n118 = Not(x=w352) -> (.not. x?=w349:bool)
        n119 = And(x="Automatic 3", y=w349) -> (x .and. y?=w351:bool)
        n120 = call-poly <vilib>:"PID Advanced.vi"("setpoint"=w345, "auto? (T)"=w351, "manual control"="MV: 3", "process variable"=w346, "alpha"=10.0, "PID gains"=w353, "dt (s)"=w354, "reinitialize? (F)"=w350) -> ("output"=w343:dbl)  [unwired: 6 in, 1 out]
      }
      frame True {
        w364 = 10000 ("sample length")
        # "Buffering data for parameters estimation"
        n121 = call <vilib>:"Data Queue PtByPt.vi"("initial queue element"=w358, "initialize"=w357, "sample length"=w364, "input data point"=w358) -> ("Current Queue"=→"Control Output 3":dbl[])  [unwired: 3 in, 4 out]
        n122 = Select(t=0.0, s=w357, f="Excitation 3") -> (s? t:f=w362:dbl)
        n123 = Add(x=w361, y=w362) -> (x+y=w359:dbl)
        n124 = call <vilib>:"Data Queue PtByPt.vi"("initial queue element"=w359, "initialize"=w357, "sample length"=w364, "input data point"=w359) -> ("Current Queue"=→"Measurement 3":dbl[])  [unwired: 3 in, 4 out]
      }
    }
    n125 = feedback-in #6(w292, w334) -> ()
    n126 = Greater?(x=w285, y="M-10") -> ()  [unwired: 1 out]
    n127 = Add(x=w316, y=w304) -> (x+y=w305:dbl)
    n128 = Subtract(x=w316, y=w304) -> (x-y=w303:dbl)
    n129 = Equal?(x=w314, y=w292) -> (x = y?=w311:bool)
    n130 = Greater?(x=w292, y=w314) -> (0:w310:bool)
    n131 = Select(t=w315, s=w311, f=w310) -> (s? t:f=w290:bool)
    "PWM Output 3" <- w290
    n132 = call "Plant System.vi"("Integrator ?"=w333, "Plant Input"=w292, "dt (s)"=w287, "process parameters"=w331) -> ("Plant Output"=w332:dbl)  [unwired: 11 in]
    n133 = Increment(x="Set Point 3") -> (x+1=w309:dbl)
    n134 = Decrement(x="Set Point 3") -> (x-1=w308:dbl)
    n135 = Select(t=w305, s=w290, f=w303) -> (s? t:f=w318:dbl)
    n136 = Select(t=w309, s=w290, f=w308) -> (s? t:f=w307:dbl)
    n137 = Not(x=w290) -> (.not. x?=w289:bool)
    n138 = call-poly <vilib>:"DAQmx Create Virtual Channel.vi"("lines"=tag "cDAQ1Mod8/port0/line6", "line grouping"=w296) -> ("task out"=w298:refnum<k21>, "error out"=w297:errorcluster)  [unwired: 12 in]
    n139 = call-poly <vilib>:"DAQmx Create Virtual Channel.vi"("lines"=tag "cDAQ1Mod7/port0/line5", "line grouping"=w278) -> ("task out"=w280:refnum<k21>, "error out"=w279:errorcluster)  [unwired: 12 in]
    n140 = Build Array(w285, "Set Point 3", w307) -> (w306:dbl[])
    n141 = Initialize Array("INLET 10 ON/OFF", 1 ("dimension size")) -> (w275:bool[])
    n142 = Initialize Array(w289, 1 ("dimension size")) -> (w293:bool[])
    n143 = local write "MV: 3"(w292) -> ()
    n144 = Add(x=w313, y=w316) -> (x+y=w317:dbl)
    n145 = Build Array(w306) -> (→"Real time Data 3":dbl[][])
    n146 = call-poly <vilib>:"DAQmx Write.vi"("task/channels in"=w298, "auto start"=TRUE, "data"=w293, "error in"=w297) -> ("task out"=w300:refnum<k21>, "error out"=w301:errorcluster)  [unwired: 9 in, 1 out]
    n147 = call-poly <vilib>:"DAQmx Write.vi"("task/channels in"=w280, "auto start"=TRUE, "data"=w275, "error in"=w279) -> ("task out"=w282:refnum<k21>, "error out"=w283:errorcluster)  [unwired: 9 in, 1 out]
    n148 = call <vilib>:"DAQmx Clear Task.vi"("task in"=w300, "error in"=w301) -> ("error out"=w295:errorcluster)  [unwired: 13 in]
    n149 = call <vilib>:"DAQmx Clear Task.vi"("task in"=w282, "error in"=w283) -> ("error out"=w277:errorcluster)  [unwired: 13 in]
    n150 = call <vilib>:"Simple Error Handler.vi"("error in (no error)"=w295) -> ()  [unwired: 4 in, 5 out]
    n151 = call <vilib>:"Simple Error Handler.vi"("error in (no error)"=w277) -> ()  [unwired: 4 in, 5 out]
  }
  n152 = while {
    shift-left: 0.0 ("Plant Output") -> [w429]
    shift-right: [w424] -> _
    tunnel: w24 -> [_]
    shift-right: [w410] -> _
    shift-left: 0.01 -> [w408]
    shift-right: [w382] -> _
    shift-left: TRUE -> [w407]
    shift-right: [w384] -> _
    shift-left: w21 -> [w406]
    shift-right: [w409] -> _
    shift-left: w21 -> [w405]
    tunnel: [w379] -> w20
    tunnel: w1 -> [w365]
    stop <- "Stop 5" stop-if-true
    w370 = 1 items=["one channel for each line", "one channel for all lines"] ("line grouping")
    w379 = 0.05 ("Sampling Time dt (s)")
    w388 = 1 items=["one channel for each line", "one channel for all lines"] ("line grouping")
    w396 = 0.5 ("x")
    w423 = T7 {"static gain"=2.5, "lag (s)"=2.5, "deadtime (s)"=0.01, "load"=0.0, "deadband"=0.0, "sensor noise"=0.0, "initial PV"=30.0, "plant noise"=0.0}  # Process parameters
    w425 = FALSE  # Integrator ?
    # "C."
    # "Inlet 11"
    # "Exhaust 8"
    # "B."
    # "A."
    # "A.Output to PWM Logic \nB. Simulated Plant\nC. Draw Chart"
    # "Main PID Loop Control"
    n153 = Multiply(x=w379, y=1000.0) -> (x*y=w422:dbl)
    n154 = Not(x="Autotune 5") -> (.not. x?=w426:bool)
    n155 = feedback #7() -> (w431:bool)  [unwired: 1 in]
    n156 = feedback-in #7("Autotune 5") -> ()
    n157 = Wait Until Next ms Multiple(millisecond multiple=w422) -> ()  [unwired: 1 out]
    n158 = Exclusive Or(1:w431, 2:"Autotune 5") -> (0:w430:bool)
    n159 = feedback #8() -> (w428:dbl)  [unwired: 1 in]
    n160 = Multiply(x=w365, y=-1000.0) -> (x*y=w412:dynamicdata)
    n161 = call <vilib>:"Median PtByPt.vi"("sample length"="Median sample length 14", "x"=w412) -> ("median"=w411:dbl)  [unwired: 2 in, 1 out]
    n162 = Square(x=w411) -> (x^2=w419:dbl)
    n163 = Multiply(x=w411, y=-39.646) -> (x*y=w415:dbl)
    n164 = Multiply(x=w419, y=0.2324) -> (x*y=w416:dbl)
    n165 = Add(x=w415, y=w416) -> (x+y=w414:dbl)
    n166 = Add(x=1678.0, y=w414) -> (x+y=w377:dbl)
    n167 = case shown="False" "Autotune 5" {
      tunnel: w379 -> [w446 _]
      tunnel: [w435 w451] -> w384
      tunnel: w429 -> [_ w450]
      tunnel: "PID Gains 5" -> [w445 _]
      tunnel: "Reinitialize 5" -> [w442 _]
      tunnel: w430 -> [w444 w449]
      tunnel: w428 -> [_ w453]
      tunnel: w377 -> [w438 _]
      tunnel: "Set Point 5" -> [w437 _]
      frame False {
        # "This code is to have 'bumpless' transfer from autotuning"
        n168 = Not(x=w444) -> (.not. x?=w441:bool)
        n169 = And(x="Automatic 5", y=w441) -> (x .and. y?=w443:bool)
        n170 = call-poly <vilib>:"PID Advanced.vi"("setpoint"=w437, "auto? (T)"=w443, "manual control"="MV: 5", "process variable"=w438, "alpha"=10.0, "PID gains"=w445, "dt (s)"=w446, "reinitialize? (F)"=w442) -> ("output"=w435:dbl)  [unwired: 6 in, 1 out]
      }
      frame True {
        w456 = 10000 ("sample length")
        # "Buffering data for parameters estimation"
        n171 = call <vilib>:"Data Queue PtByPt.vi"("initial queue element"=w450, "initialize"=w449, "sample length"=w456, "input data point"=w450) -> ("Current Queue"=→"Control Output 5":dbl[])  [unwired: 3 in, 4 out]
        n172 = Select(t=0.0, s=w449, f="Excitation 5") -> (s? t:f=w454:dbl)
        n173 = Add(x=w453, y=w454) -> (x+y=w451:dbl)
        n174 = call <vilib>:"Data Queue PtByPt.vi"("initial queue element"=w451, "initialize"=w449, "sample length"=w456, "input data point"=w451) -> ("Current Queue"=→"Measurement 5":dbl[])  [unwired: 3 in, 4 out]
      }
    }
    n175 = feedback-in #8(w384, w426) -> ()
    n176 = Greater?(x=w377, y="M-8") -> ()  [unwired: 1 out]
    n177 = Add(x=w408, y=w396) -> (x+y=w397:dbl)
    n178 = Subtract(x=w408, y=w396) -> (x-y=w395:dbl)
    n179 = Equal?(x=w406, y=w384) -> (x = y?=w403:bool)
    n180 = Greater?(x=w384, y=w406) -> (0:w402:bool)
    n181 = Select(t=w407, s=w403, f=w402) -> (s? t:f=w382:bool)
    "PWM Output 5" <- w382
    n182 = call "Plant System.vi"("Integrator ?"=w425, "Plant Input"=w384, "dt (s)"=w379, "process parameters"=w423) -> ("Plant Output"=w424:dbl)  [unwired: 11 in]
    n183 = Increment(x="Set Point 5") -> (x+1=w401:dbl)
    n184 = Decrement(x="Set Point 5") -> (x-1=w400:dbl)
    n185 = Select(t=w397, s=w382, f=w395) -> (s? t:f=w410:dbl)
    n186 = Select(t=w401, s=w382, f=w400) -> (s? t:f=w399:dbl)
    n187 = Not(x=w382) -> (.not. x?=w381:bool)
    n188 = call-poly <vilib>:"DAQmx Create Virtual Channel.vi"("lines"=tag "cDAQ1Mod8/port0/line3", "line grouping"=w388) -> ("task out"=w390:refnum<k21>, "error out"=w389:errorcluster)  [unwired: 12 in]
    n189 = call-poly <vilib>:"DAQmx Create Virtual Channel.vi"("lines"=tag "cDAQ1Mod7/port0/line2", "line grouping"=w370) -> ("task out"=w372:refnum<k21>, "error out"=w371:errorcluster)  [unwired: 12 in]
    n190 = Build Array(w377, "Set Point 5", w399) -> (w398:dbl[])
    n191 = Initialize Array("INLET 8 ON/OFF 2", 1 ("dimension size")) -> (w367:bool[])
    n192 = Initialize Array(w381, 1 ("dimension size")) -> (w385:bool[])
    n193 = local write "MV: 5"(w384) -> ()
    n194 = Add(x=w405, y=w408) -> (x+y=w409:dbl)
    n195 = Build Array(w398) -> (→"Real time Data 5":dbl[][])
    n196 = call-poly <vilib>:"DAQmx Write.vi"("task/channels in"=w390, "auto start"=TRUE, "data"=w385, "error in"=w389) -> ("task out"=w392:refnum<k21>, "error out"=w393:errorcluster)  [unwired: 9 in, 1 out]
    n197 = call-poly <vilib>:"DAQmx Write.vi"("task/channels in"=w372, "auto start"=TRUE, "data"=w367, "error in"=w371) -> ("task out"=w374:refnum<k21>, "error out"=w375:errorcluster)  [unwired: 9 in, 1 out]
    n198 = call <vilib>:"DAQmx Clear Task.vi"("task in"=w392, "error in"=w393) -> ("error out"=w387:errorcluster)  [unwired: 13 in]
    n199 = call <vilib>:"DAQmx Clear Task.vi"("task in"=w374, "error in"=w375) -> ("error out"=w369:errorcluster)  [unwired: 13 in]
    n200 = call <vilib>:"Simple Error Handler.vi"("error in (no error)"=w387) -> ()  [unwired: 4 in, 5 out]
    n201 = call <vilib>:"Simple Error Handler.vi"("error in (no error)"=w369) -> ()  [unwired: 4 in, 5 out]
  }
  n202 = while {
    shift-left: 0.0 ("Plant Output") -> [w521]
    shift-right: [w516] -> _
    tunnel: w42 -> [_]
    shift-right: [w502] -> _
    shift-left: 0.01 -> [w500]
    shift-right: [w474] -> _
    shift-left: TRUE -> [w499]
    shift-right: [w476] -> _
    shift-left: w39 -> [w498]
    shift-right: [w501] -> _
    shift-left: w39 -> [w497]
    tunnel: [w471] -> w38
    tunnel: w1 -> [w457]
    stop <- "Stop 2" stop-if-true
    w462 = 1 items=["one channel for each line", "one channel for all lines"] ("line grouping")
    w471 = 0.05 ("Sampling Time dt (s)")
    w480 = 1 items=["one channel for each line", "one channel for all lines"] ("line grouping")
    w488 = 0.5 ("x")
    w515 = T7 {"static gain"=2.5, "lag (s)"=2.5, "deadtime (s)"=0.01, "load"=0.0, "deadband"=0.0, "sensor noise"=0.0, "initial PV"=30.0, "plant noise"=0.0}  # Process parameters
    w517 = FALSE  # Integrator ?
    # "C."
    # "Inlet 11"
    # "Exhaust 12"
    # "B."
    # "A."
    # "A.Output to PWM Logic \nB. Simulated Plant\nC. Draw Chart"
    # "Main PID Loop Control"
    n203 = Multiply(x=w471, y=1000.0) -> (x*y=w514:dbl)
    n204 = Not(x="Autotune 2") -> (.not. x?=w518:bool)
    n205 = feedback #9() -> (w523:bool)  [unwired: 1 in]
    n206 = feedback-in #9("Autotune 2") -> ()
    n207 = Wait Until Next ms Multiple(millisecond multiple=w514) -> ()  [unwired: 1 out]
    n208 = Exclusive Or(1:w523, 2:"Autotune 2") -> (0:w522:bool)
    n209 = feedback #10() -> (w520:dbl)  [unwired: 1 in]
    n210 = Multiply(x=w457, y=-1000.0) -> (x*y=w504:dynamicdata)
    n211 = call <vilib>:"Median PtByPt.vi"("sample length"="Median sample length 12", "x"=w504) -> ("median"=w503:dbl)  [unwired: 2 in, 1 out]
    n212 = Square(x=w503) -> (x^2=w511:dbl)
    n213 = Multiply(x=w503, y=-39.646) -> (x*y=w507:dbl)
    n214 = Multiply(x=w511, y=0.2324) -> (x*y=w508:dbl)
    n215 = Add(x=w507, y=w508) -> (x+y=w506:dbl)
    n216 = Add(x=1678.0, y=w506) -> (x+y=w469:dbl)
    n217 = case shown="False" "Autotune 2" {
      tunnel: w471 -> [w538 _]
      tunnel: [w527 w543] -> w476
      tunnel: w521 -> [_ w542]
      tunnel: "PID Gains 2" -> [w537 _]
      tunnel: "Reinitialize 2" -> [w534 _]
      tunnel: w522 -> [w536 w541]
      tunnel: w520 -> [_ w545]
      tunnel: w469 -> [w530 _]
      tunnel: "Set Point 2" -> [w529 _]
      frame False {
        # "This code is to have 'bumpless' transfer from autotuning"
        n218 = Not(x=w536) -> (.not. x?=w533:bool)
        n219 = And(x="Automatic 2", y=w533) -> (x .and. y?=w535:bool)
        n220 = call-poly <vilib>:"PID Advanced.vi"("setpoint"=w529, "auto? (T)"=w535, "manual control"="MV: 2", "process variable"=w530, "alpha"=10.0, "PID gains"=w537, "dt (s)"=w538, "reinitialize? (F)"=w534) -> ("output"=w527:dbl)  [unwired: 6 in, 1 out]
      }
      frame True {
        w548 = 10000 ("sample length")
        # "Buffering data for parameters estimation"
        n221 = call <vilib>:"Data Queue PtByPt.vi"("initial queue element"=w542, "initialize"=w541, "sample length"=w548, "input data point"=w542) -> ("Current Queue"=→"Control Output 2":dbl[])  [unwired: 3 in, 4 out]
        n222 = Select(t=0.0, s=w541, f="Excitation 2") -> (s? t:f=w546:dbl)
        n223 = Add(x=w545, y=w546) -> (x+y=w543:dbl)
        n224 = call <vilib>:"Data Queue PtByPt.vi"("initial queue element"=w543, "initialize"=w541, "sample length"=w548, "input data point"=w543) -> ("Current Queue"=→"Measurement 2":dbl[])  [unwired: 3 in, 4 out]
      }
    }
    n225 = feedback-in #10(w476, w518) -> ()
    n226 = Greater?(x=w469, y="M-12") -> ()  [unwired: 1 out]
    n227 = Add(x=w500, y=w488) -> (x+y=w489:dbl)
    n228 = Subtract(x=w500, y=w488) -> (x-y=w487:dbl)
    n229 = Equal?(x=w498, y=w476) -> (x = y?=w495:bool)
    n230 = Greater?(x=w476, y=w498) -> (0:w494:bool)
    n231 = Select(t=w499, s=w495, f=w494) -> (s? t:f=w474:bool)
    "PWM Output 2" <- w474
    n232 = call "Plant System.vi"("Integrator ?"=w517, "Plant Input"=w476, "dt (s)"=w471, "process parameters"=w515) -> ("Plant Output"=w516:dbl)  [unwired: 11 in]
    n233 = Increment(x="Set Point 2") -> (x+1=w493:dbl)
    n234 = Decrement(x="Set Point 2") -> (x-1=w492:dbl)
    n235 = Select(t=w489, s=w474, f=w487) -> (s? t:f=w502:dbl)
    n236 = Select(t=w493, s=w474, f=w492) -> (s? t:f=w491:dbl)
    n237 = Not(x=w474) -> (.not. x?=w473:bool)
    n238 = call-poly <vilib>:"DAQmx Create Virtual Channel.vi"("lines"=tag "cDAQ1Mod8/port0/line2", "line grouping"=w480) -> ("task out"=w482:refnum<k21>, "error out"=w481:errorcluster)  [unwired: 12 in]
    n239 = call-poly <vilib>:"DAQmx Create Virtual Channel.vi"("lines"=tag "cDAQ1Mod7/port0/line1", "line grouping"=w462) -> ("task out"=w464:refnum<k21>, "error out"=w463:errorcluster)  [unwired: 12 in]
    n240 = Build Array(w469, "Set Point 2", w491) -> (w490:dbl[])
    n241 = Initialize Array("INLET 12 ON/OFF", 1 ("dimension size")) -> (w459:bool[])
    n242 = Initialize Array(w473, 1 ("dimension size")) -> (w477:bool[])
    n243 = local write "MV: 2"(w476) -> ()
    n244 = Add(x=w497, y=w500) -> (x+y=w501:dbl)
    n245 = Build Array(w490) -> (→"Real time Data 2":dbl[][])
    n246 = call-poly <vilib>:"DAQmx Write.vi"("task/channels in"=w482, "auto start"=TRUE, "data"=w477, "error in"=w481) -> ("task out"=w484:refnum<k21>, "error out"=w485:errorcluster)  [unwired: 9 in, 1 out]
    n247 = call-poly <vilib>:"DAQmx Write.vi"("task/channels in"=w464, "auto start"=TRUE, "data"=w459, "error in"=w463) -> ("task out"=w466:refnum<k21>, "error out"=w467:errorcluster)  [unwired: 9 in, 1 out]
    n248 = call <vilib>:"DAQmx Clear Task.vi"("task in"=w484, "error in"=w485) -> ("error out"=w479:errorcluster)  [unwired: 13 in]
    n249 = call <vilib>:"DAQmx Clear Task.vi"("task in"=w466, "error in"=w467) -> ("error out"=w461:errorcluster)  [unwired: 13 in]
    n250 = call <vilib>:"Simple Error Handler.vi"("error in (no error)"=w479) -> ()  [unwired: 4 in, 5 out]
    n251 = call <vilib>:"Simple Error Handler.vi"("error in (no error)"=w461) -> ()  [unwired: 4 in, 5 out]
  }
  n252 = while {
    shift-left: 0.0 ("Plant Output") -> [w614]
    shift-right: [w609] -> _
    tunnel: w87 -> [_]
    shift-right: [w595] -> _
    shift-left: 0.01 -> [w593]
    shift-right: [w567] -> _
    shift-left: TRUE -> [w592]
    shift-right: [w569] -> _
    shift-left: w84 -> [w591]
    shift-right: [w594] -> _
    shift-left: w84 -> [w590]
    tunnel: [w564] -> w83
    tunnel: [w561] -> w46
    tunnel: w1 -> [w549]
    stop <- "Stop" stop-if-true
    w554 = 1 items=["one channel for each line", "one channel for all lines"] ("line grouping")
    w564 = 0.05 ("Sampling Time dt (s)")
    w573 = 1 items=["one channel for each line", "one channel for all lines"] ("line grouping")
    w581 = 0.5 ("x")
    w608 = T7 {"static gain"=2.5, "lag (s)"=2.5, "deadtime (s)"=0.01, "load"=0.0, "deadband"=0.0, "sensor noise"=0.0, "initial PV"=30.0, "plant noise"=0.0}  # Process parameters
    w610 = FALSE  # Integrator ?
    # "C."
    # "Inlet 11"
    # "Exhaust 11"
    # "B."
    # "A."
    # "A.Output to PWM Logic \nB. Simulated Plant\nC. Draw Chart"
    # "Main PID Loop Control"
    n253 = Multiply(x=w564, y=1000.0) -> (x*y=w607:dbl)
    n254 = Not(x="Autotune") -> (.not. x?=w611:bool)
    n255 = feedback #11() -> (w616:bool)  [unwired: 1 in]
    n256 = feedback-in #11("Autotune") -> ()
    n257 = Wait Until Next ms Multiple(millisecond multiple=w607) -> ()  [unwired: 1 out]
    n258 = Exclusive Or(1:w616, 2:"Autotune") -> (0:w615:bool)
    n259 = feedback #12() -> (w613:dbl)  [unwired: 1 in]
    n260 = Multiply(x=w549, y=-1000.0) -> (x*y=w597:dynamicdata)
    n261 = call <vilib>:"Median PtByPt.vi"("sample length"="Median sample length", "x"=w597) -> ("median"=w596:dbl)  [unwired: 2 in, 1 out]
    n262 = Square(x=w596) -> (x^2=w604:dbl)
    n263 = Multiply(x=w596, y=-39.646) -> (x*y=w600:dbl)
    n264 = Multiply(x=w604, y=0.2324) -> (x*y=w601:dbl)
    n265 = Add(x=w600, y=w601) -> (x+y=w599:dbl)
    n266 = Add(x=1678.0, y=w599) -> (x+y=w562:dbl)
    n267 = case shown="False" "Autotune" {
      tunnel: w564 -> [w631 _]
      tunnel: [w620 w636] -> w569
      tunnel: w614 -> [_ w635]
      tunnel: "PID Gains" -> [w630 _]
      tunnel: "Reinitialize" -> [w627 _]
      tunnel: w615 -> [w629 w634]
      tunnel: w613 -> [_ w638]
      tunnel: w562 -> [w623 _]
      tunnel: "Set Point" -> [w622 _]
      frame False {
        # "This code is to have 'bumpless' transfer from autotuning"
        n268 = Not(x=w629) -> (.not. x?=w626:bool)
        n269 = And(x="Automatic", y=w626) -> (x .and. y?=w628:bool)
        n270 = call-poly <vilib>:"PID Advanced.vi"("setpoint"=w622, "auto? (T)"=w628, "manual control"="MV:", "process variable"=w623, "alpha"=10.0, "PID gains"=w630, "dt (s)"=w631, "reinitialize? (F)"=w627) -> ("output"=w620:dbl)  [unwired: 6 in, 1 out]
      }
      frame True {
        w641 = 10000 ("sample length")
        # "Buffering data for parameters estimation"
        n271 = call <vilib>:"Data Queue PtByPt.vi"("initial queue element"=w635, "initialize"=w634, "sample length"=w641, "input data point"=w635) -> ("Current Queue"=→"Control Output":dbl[])  [unwired: 3 in, 4 out]
        n272 = Select(t=0.0, s=w634, f="Excitation") -> (s? t:f=w639:dbl)
        n273 = Add(x=w638, y=w639) -> (x+y=w636:dbl)
        n274 = call <vilib>:"Data Queue PtByPt.vi"("initial queue element"=w636, "initialize"=w634, "sample length"=w641, "input data point"=w636) -> ("Current Queue"=→"Measurement":dbl[])  [unwired: 3 in, 4 out]
      }
    }
    n275 = feedback-in #12(w569, w611) -> ()
    n276 = Greater?(x=w562, y="M-11") -> (0:w561:bool)
    "?" <- w561
    n277 = Add(x=w593, y=w581) -> (x+y=w582:dbl)
    n278 = Subtract(x=w593, y=w581) -> (x-y=w580:dbl)
    n279 = Equal?(x=w591, y=w569) -> (x = y?=w588:bool)
    n280 = Greater?(x=w569, y=w591) -> (0:w587:bool)
    n281 = Select(t=w592, s=w588, f=w587) -> (s? t:f=w567:bool)
    "PWM Output" <- w567
    n282 = call "Plant System.vi"("Integrator ?"=w610, "Plant Input"=w569, "dt (s)"=w564, "process parameters"=w608) -> ("Plant Output"=w609:dbl)  [unwired: 11 in]
    n283 = Increment(x="Set Point") -> (x+1=w586:dbl)
    n284 = Decrement(x="Set Point") -> (x-1=w585:dbl)
    n285 = Select(t=w582, s=w567, f=w580) -> (s? t:f=w595:dbl)
    n286 = Select(t=w586, s=w567, f=w585) -> (s? t:f=w584:dbl)
    n287 = Not(x=w567) -> (.not. x?=w566:bool)
    n288 = call-poly <vilib>:"DAQmx Create Virtual Channel.vi"("lines"=tag "cDAQ1Mod1/port0/line2", "line grouping"=w573) -> ("task out"=w575:refnum<k21>, "error out"=w574:errorcluster)  [unwired: 12 in]
    n289 = call-poly <vilib>:"DAQmx Create Virtual Channel.vi"("lines"=tag "cDAQ1Mod2/port0/line2", "line grouping"=w554) -> ("task out"=w556:refnum<k21>, "error out"=w555:errorcluster)  [unwired: 12 in]
    n290 = Build Array(w562, "Set Point", w584) -> (w583:dbl[])
    n291 = Initialize Array("INLET", 1 ("dimension size")) -> (w551:bool[])
    n292 = Initialize Array(w566, 1 ("dimension size")) -> (w570:bool[])
    n293 = local write "MV:"(w569) -> ()
    n294 = Add(x=w590, y=w593) -> (x+y=w594:dbl)
    n295 = Build Array(w583) -> (→"Real time Data":dbl[][])
    n296 = call-poly <vilib>:"DAQmx Write.vi"("task/channels in"=w575, "auto start"=TRUE, "data"=w570, "error in"=w574) -> ("task out"=w577:refnum<k21>, "error out"=w578:errorcluster)  [unwired: 9 in, 1 out]
    n297 = call-poly <vilib>:"DAQmx Write.vi"("task/channels in"=w556, "auto start"=TRUE, "data"=w551, "error in"=w555) -> ("task out"=w558:refnum<k21>, "error out"=w559:errorcluster)  [unwired: 9 in, 1 out]
    n298 = call <vilib>:"DAQmx Clear Task.vi"("task in"=w577, "error in"=w578) -> ("error out"=w572:errorcluster)  [unwired: 13 in]
    n299 = call <vilib>:"DAQmx Clear Task.vi"("task in"=w558, "error in"=w559) -> ("error out"=w553:errorcluster)  [unwired: 13 in]
    n300 = call <vilib>:"Simple Error Handler.vi"("error in (no error)"=w572) -> ()  [unwired: 4 in, 5 out]
    n301 = call <vilib>:"Simple Error Handler.vi"("error in (no error)"=w553) -> ()  [unwired: 4 in, 5 out]
  }
  n302 = local write "Stop 6"(w18) -> ()
  n303 = local write "Stop 4"(w30) -> ()
  n304 = local write "Stop 3"(w36) -> ()
  n305 = local write "Stop 5"(w24) -> ()
  n306 = local write "Stop 2"(w42) -> ()
  n307 = stacked-sequence {
    tunnel: [_ w647] -> w54
    tunnel: [_ w646] -> w53
    frame #0 {
      w642 = 0
      w643 = FALSE
      w644 = ""
      # "Initialize Indicators"
      "Connected" <- w643
      "Start Time Text" <- w644
      "Stop Time Text" <- w644
      "Elapsed Time Text" <- w644
      "HostFrameCount" <- w642
      "Running" <- w643
      "Loop Iter" <- w642
      "PnoData" <- w643
    }
    frame #1 {
      # "Connect To Tracker"
      # "2. Initialize Tracker Connection"
      n308 = call <instrlib>:"PDI initialize.vi"() -> ("error out"=w646:errorcluster, "Connected"=w645:bool, "pDev"=w647:u32)  [unwired: 1 in, 4 out]
      n309 = local write "Connected"(w645) -> ()
    }
  }
  n310 = local write "Stop"(w87) -> ()
  n311 = call-poly "VISA Configure Serial Port"("VISA resource name"="COM Port-Sensor 1") -> ("VISA resource name out"=w78:refnum<visa-resource-name>, "error out"=w77:errorcluster)  [unwired: 9 in, 4 out]
  n312 = call-poly "VISA Configure Serial Port"("VISA resource name"="COM Port-Sensor 2") -> ("VISA resource name out"=w73:refnum<visa-resource-name>, "error out"=w72:errorcluster)  [unwired: 9 in, 4 out]
  n313 = while {
    tunnel: w18 -> [_]
    tunnel: w14 -> [w651]
    stop <- w661 stop-if-true
    # "If dT and deadtime have similar values, the identification could evaluate deadtime as zero and this generates proportional gain equal to Inf. This code avoid gain changes in this situations."
    # "Autotuning Loop"
    n314 = local read "Control Output 6"() -> (w663:dbl[])
    n315 = local read "Measurement 6"() -> (w662:dbl[])
    n316 = case shown="\"Chien-Hrones-Reswick\"" "Control 6" {
      tunnel: w663 -> [w672 w680 w689 w698]
      tunnel: w662 -> [w671 w679 w688 w697]
      tunnel: [w670 w678 w687 w696] -> w650
      tunnel: [w669 w677 w686 w695] -> w649
      tunnel: w651 -> [w668 w676 w685 w694]
      tunnel: [w667 w675 w684 w693] -> w648
      tunnel: [w666 w674 w683 w692] -> w653
      tunnel: "Type of controller 6" -> [w665 w673 w682 w691]
      frame "Ziegler-Nichols", Default {
        n317 = call-poly <vilib>:"PID Autotuning Design.vi"("Ziegler-Nichols Speed"="Ziegler-Nichols speed 6", "Type of Controller"=w665, "dt (s)"=w668, "Response signal"=w671, "Stimulus signal"=w672) -> ("PID gains"=w666:T2, "response operating point"=w669:dbl, "stimulus operating point"=w670:dbl, "Plant Parameters"=w667:T4)  [unwired: 3 in]
      }
      frame "Cohen-Coon" {
        n318 = call-poly <vilib>:"PID Autotuning Design.vi"("Type of Controller"=w673, "dt (s)"=w676, "Response signal"=w679, "Stimulus signal"=w680) -> ("PID gains"=w674:T2, "response offset"=w677:dbl, "stimulus offset"=w678:dbl, "Plant Parameters"=w675:T4)  [unwired: 4 in]
      }
      frame "Chien-Hrones-Reswick" {
        n319 = call-poly <vilib>:"PID Autotuning Design.vi"("Tuning specifications"="Tuning specifications 6", "Type of Controller"=w682, "dt (s)"=w685, "Response signal"=w688, "Stimulus signal"=w689) -> ("PID gains"=w683:T2, "response offset"=w686:dbl, "stimulus offset"=w687:dbl, "Plant Parameters"=w684:T4)  [unwired: 3 in]
      }
      frame "Internal Model Control" {
        n320 = call-poly <vilib>:"PID Autotuning Design.vi"("Desired Time Constant (tau_c)"="Multiplicative factor 6", "Type of Controller"=w691, "dt (s)"=w694, "Response signal"=w697, "Stimulus signal"=w698) -> ("PID gains"=w692:T2, "response offset"=w695:dbl, "stimulus offset"=w696:dbl, "Plant Parameters"=w693:T4)  [unwired: 3 in]
      }
    }
    "Stimulus operating point 6" <- w650
    "Response operating point 6" <- w649
    "Identified Plant Parameters 6" <- w648
    n321 = Unbundle(w653) -> ("proportional gain (Kc)"=w656:dbl)  [unwired: 2 out]
    n322 = Equal?(x=w656, y=inf) -> (x = y?=w655:bool)
    n323 = feedback #13() -> (w654:T2)  [unwired: 1 in]
    n324 = Select(t=w654, s=w655, f=w653) -> (s? t:f=w652:T2)
    "Tuned PID gains 6" <- w652
    n325 = feedback-in #13(w652) -> ()
    n326 = case shown="True" "Accept gain 6" {
      tunnel: w652 -> [_ w699]
      frame False {
      }
      frame True {
        n327 = local write "PID Gains 6"(w699) -> ()
      }
    }
    n328 = local read "Stop 6"() -> (w661:bool)
  }
  n329 = while {
    tunnel: w30 -> [_]
    tunnel: w26 -> [w703]
    stop <- w713 stop-if-true
    # "If dT and deadtime have similar values, the identification could evaluate deadtime as zero and this generates proportional gain equal to Inf. This code avoid gain changes in this situations."
    # "Autotuning Loop"
    n330 = local read "Control Output 4"() -> (w715:dbl[])
    n331 = local read "Measurement 4"() -> (w714:dbl[])
    n332 = case shown="\"Chien-Hrones-Reswick\"" "Control 4" {
      tunnel: w715 -> [w724 w732 w741 w750]
      tunnel: w714 -> [w723 w731 w740 w749]
      tunnel: [w722 w730 w739 w748] -> w702
      tunnel: [w721 w729 w738 w747] -> w701
      tunnel: w703 -> [w720 w728 w737 w746]
      tunnel: [w719 w727 w736 w745] -> w700
      tunnel: [w718 w726 w735 w744] -> w705
      tunnel: "Type of controller 4" -> [w717 w725 w734 w743]
      frame "Ziegler-Nichols", Default {
        n333 = call-poly <vilib>:"PID Autotuning Design.vi"("Ziegler-Nichols Speed"="Ziegler-Nichols speed 4", "Type of Controller"=w717, "dt (s)"=w720, "Response signal"=w723, "Stimulus signal"=w724) -> ("PID gains"=w718:T2, "response operating point"=w721:dbl, "stimulus operating point"=w722:dbl, "Plant Parameters"=w719:T4)  [unwired: 3 in]
      }
      frame "Cohen-Coon" {
        n334 = call-poly <vilib>:"PID Autotuning Design.vi"("Type of Controller"=w725, "dt (s)"=w728, "Response signal"=w731, "Stimulus signal"=w732) -> ("PID gains"=w726:T2, "response offset"=w729:dbl, "stimulus offset"=w730:dbl, "Plant Parameters"=w727:T4)  [unwired: 4 in]
      }
      frame "Chien-Hrones-Reswick" {
        n335 = call-poly <vilib>:"PID Autotuning Design.vi"("Tuning specifications"="Tuning specifications 4", "Type of Controller"=w734, "dt (s)"=w737, "Response signal"=w740, "Stimulus signal"=w741) -> ("PID gains"=w735:T2, "response offset"=w738:dbl, "stimulus offset"=w739:dbl, "Plant Parameters"=w736:T4)  [unwired: 3 in]
      }
      frame "Internal Model Control" {
        n336 = call-poly <vilib>:"PID Autotuning Design.vi"("Desired Time Constant (tau_c)"="Multiplicative factor 4", "Type of Controller"=w743, "dt (s)"=w746, "Response signal"=w749, "Stimulus signal"=w750) -> ("PID gains"=w744:T2, "response offset"=w747:dbl, "stimulus offset"=w748:dbl, "Plant Parameters"=w745:T4)  [unwired: 3 in]
      }
    }
    "Stimulus operating point 4" <- w702
    "Response operating point 4" <- w701
    "Identified Plant Parameters 4" <- w700
    n337 = Unbundle(w705) -> ("proportional gain (Kc)"=w708:dbl)  [unwired: 2 out]
    n338 = Equal?(x=w708, y=inf) -> (x = y?=w707:bool)
    n339 = feedback #14() -> (w706:T2)  [unwired: 1 in]
    n340 = Select(t=w706, s=w707, f=w705) -> (s? t:f=w704:T2)
    "Tuned PID gains 4" <- w704
    n341 = feedback-in #14(w704) -> ()
    n342 = case shown="True" "Accept gain 4" {
      tunnel: w704 -> [_ w751]
      frame False {
      }
      frame True {
        n343 = local write "PID Gains 4"(w751) -> ()
      }
    }
    n344 = local read "Stop 4"() -> (w713:bool)
  }
  n345 = while {
    tunnel: w36 -> [_]
    tunnel: w32 -> [w755]
    stop <- w765 stop-if-true
    # "If dT and deadtime have similar values, the identification could evaluate deadtime as zero and this generates proportional gain equal to Inf. This code avoid gain changes in this situations."
    # "Autotuning Loop"
    n346 = local read "Control Output 3"() -> (w767:dbl[])
    n347 = local read "Measurement 3"() -> (w766:dbl[])
    n348 = case shown="\"Chien-Hrones-Reswick\"" "Control 3" {
      tunnel: w767 -> [w776 w784 w793 w802]
      tunnel: w766 -> [w775 w783 w792 w801]
      tunnel: [w774 w782 w791 w800] -> w754
      tunnel: [w773 w781 w790 w799] -> w753
      tunnel: w755 -> [w772 w780 w789 w798]
      tunnel: [w771 w779 w788 w797] -> w752
      tunnel: [w770 w778 w787 w796] -> w757
      tunnel: "Type of controller 3" -> [w769 w777 w786 w795]
      frame "Ziegler-Nichols", Default {
        n349 = call-poly <vilib>:"PID Autotuning Design.vi"("Ziegler-Nichols Speed"="Ziegler-Nichols speed 3", "Type of Controller"=w769, "dt (s)"=w772, "Response signal"=w775, "Stimulus signal"=w776) -> ("PID gains"=w770:T2, "response operating point"=w773:dbl, "stimulus operating point"=w774:dbl, "Plant Parameters"=w771:T4)  [unwired: 3 in]
      }
      frame "Cohen-Coon" {
        n350 = call-poly <vilib>:"PID Autotuning Design.vi"("Type of Controller"=w777, "dt (s)"=w780, "Response signal"=w783, "Stimulus signal"=w784) -> ("PID gains"=w778:T2, "response offset"=w781:dbl, "stimulus offset"=w782:dbl, "Plant Parameters"=w779:T4)  [unwired: 4 in]
      }
      frame "Chien-Hrones-Reswick" {
        n351 = call-poly <vilib>:"PID Autotuning Design.vi"("Tuning specifications"="Tuning specifications 3", "Type of Controller"=w786, "dt (s)"=w789, "Response signal"=w792, "Stimulus signal"=w793) -> ("PID gains"=w787:T2, "response offset"=w790:dbl, "stimulus offset"=w791:dbl, "Plant Parameters"=w788:T4)  [unwired: 3 in]
      }
      frame "Internal Model Control" {
        n352 = call-poly <vilib>:"PID Autotuning Design.vi"("Desired Time Constant (tau_c)"="Multiplicative factor 3", "Type of Controller"=w795, "dt (s)"=w798, "Response signal"=w801, "Stimulus signal"=w802) -> ("PID gains"=w796:T2, "response offset"=w799:dbl, "stimulus offset"=w800:dbl, "Plant Parameters"=w797:T4)  [unwired: 3 in]
      }
    }
    "Stimulus operating point 3" <- w754
    "Response operating point 3" <- w753
    "Identified Plant Parameters 3" <- w752
    n353 = Unbundle(w757) -> ("proportional gain (Kc)"=w760:dbl)  [unwired: 2 out]
    n354 = Equal?(x=w760, y=inf) -> (x = y?=w759:bool)
    n355 = feedback #15() -> (w758:T2)  [unwired: 1 in]
    n356 = Select(t=w758, s=w759, f=w757) -> (s? t:f=w756:T2)
    "Tuned PID gains 3" <- w756
    n357 = feedback-in #15(w756) -> ()
    n358 = case shown="True" "Accept gain 3" {
      tunnel: w756 -> [_ w803]
      frame False {
      }
      frame True {
        n359 = local write "PID Gains 3"(w803) -> ()
      }
    }
    n360 = local read "Stop 3"() -> (w765:bool)
  }
  n361 = while {
    tunnel: w24 -> [_]
    tunnel: w20 -> [w807]
    stop <- w817 stop-if-true
    # "If dT and deadtime have similar values, the identification could evaluate deadtime as zero and this generates proportional gain equal to Inf. This code avoid gain changes in this situations."
    # "Autotuning Loop"
    n362 = local read "Control Output 5"() -> (w819:dbl[])
    n363 = local read "Measurement 5"() -> (w818:dbl[])
    n364 = case shown="\"Chien-Hrones-Reswick\"" "Control 5" {
      tunnel: w819 -> [w828 w836 w845 w854]
      tunnel: w818 -> [w827 w835 w844 w853]
      tunnel: [w826 w834 w843 w852] -> w806
      tunnel: [w825 w833 w842 w851] -> w805
      tunnel: w807 -> [w824 w832 w841 w850]
      tunnel: [w823 w831 w840 w849] -> w804
      tunnel: [w822 w830 w839 w848] -> w809
      tunnel: "Type of controller 5" -> [w821 w829 w838 w847]
      frame "Ziegler-Nichols", Default {
        n365 = call-poly <vilib>:"PID Autotuning Design.vi"("Ziegler-Nichols Speed"="Ziegler-Nichols speed 5", "Type of Controller"=w821, "dt (s)"=w824, "Response signal"=w827, "Stimulus signal"=w828) -> ("PID gains"=w822:T2, "response operating point"=w825:dbl, "stimulus operating point"=w826:dbl, "Plant Parameters"=w823:T4)  [unwired: 3 in]
      }
      frame "Cohen-Coon" {
        n366 = call-poly <vilib>:"PID Autotuning Design.vi"("Type of Controller"=w829, "dt (s)"=w832, "Response signal"=w835, "Stimulus signal"=w836) -> ("PID gains"=w830:T2, "response offset"=w833:dbl, "stimulus offset"=w834:dbl, "Plant Parameters"=w831:T4)  [unwired: 4 in]
      }
      frame "Chien-Hrones-Reswick" {
        n367 = call-poly <vilib>:"PID Autotuning Design.vi"("Tuning specifications"="Tuning specifications 5", "Type of Controller"=w838, "dt (s)"=w841, "Response signal"=w844, "Stimulus signal"=w845) -> ("PID gains"=w839:T2, "response offset"=w842:dbl, "stimulus offset"=w843:dbl, "Plant Parameters"=w840:T4)  [unwired: 3 in]
      }
      frame "Internal Model Control" {
        n368 = call-poly <vilib>:"PID Autotuning Design.vi"("Desired Time Constant (tau_c)"="Multiplicative factor 5", "Type of Controller"=w847, "dt (s)"=w850, "Response signal"=w853, "Stimulus signal"=w854) -> ("PID gains"=w848:T2, "response offset"=w851:dbl, "stimulus offset"=w852:dbl, "Plant Parameters"=w849:T4)  [unwired: 3 in]
      }
    }
    "Stimulus operating point 5" <- w806
    "Response operating point 5" <- w805
    "Identified Plant Parameters 5" <- w804
    n369 = Unbundle(w809) -> ("proportional gain (Kc)"=w812:dbl)  [unwired: 2 out]
    n370 = Equal?(x=w812, y=inf) -> (x = y?=w811:bool)
    n371 = feedback #16() -> (w810:T2)  [unwired: 1 in]
    n372 = Select(t=w810, s=w811, f=w809) -> (s? t:f=w808:T2)
    "Tuned PID gains 5" <- w808
    n373 = feedback-in #16(w808) -> ()
    n374 = case shown="True" "Accept gain 5" {
      tunnel: w808 -> [_ w855]
      frame False {
      }
      frame True {
        n375 = local write "PID Gains 5"(w855) -> ()
      }
    }
    n376 = local read "Stop 5"() -> (w817:bool)
  }
  n377 = while {
    tunnel: w42 -> [_]
    tunnel: w38 -> [w859]
    stop <- w869 stop-if-true
    # "If dT and deadtime have similar values, the identification could evaluate deadtime as zero and this generates proportional gain equal to Inf. This code avoid gain changes in this situations."
    # "Autotuning Loop"
    n378 = local read "Control Output 2"() -> (w871:dbl[])
    n379 = local read "Measurement 2"() -> (w870:dbl[])
    n380 = case shown="\"Chien-Hrones-Reswick\"" "Control 2" {
      tunnel: w871 -> [w880 w888 w897 w906]
      tunnel: w870 -> [w879 w887 w896 w905]
      tunnel: [w878 w886 w895 w904] -> w858
      tunnel: [w877 w885 w894 w903] -> w857
      tunnel: w859 -> [w876 w884 w893 w902]
      tunnel: [w875 w883 w892 w901] -> w856
      tunnel: [w874 w882 w891 w900] -> w861
      tunnel: "Type of controller 2" -> [w873 w881 w890 w899]
      frame "Ziegler-Nichols", Default {
        n381 = call-poly <vilib>:"PID Autotuning Design.vi"("Ziegler-Nichols Speed"="Ziegler-Nichols speed 2", "Type of Controller"=w873, "dt (s)"=w876, "Response signal"=w879, "Stimulus signal"=w880) -> ("PID gains"=w874:T2, "response operating point"=w877:dbl, "stimulus operating point"=w878:dbl, "Plant Parameters"=w875:T4)  [unwired: 3 in]
      }
      frame "Cohen-Coon" {
        n382 = call-poly <vilib>:"PID Autotuning Design.vi"("Type of Controller"=w881, "dt (s)"=w884, "Response signal"=w887, "Stimulus signal"=w888) -> ("PID gains"=w882:T2, "response offset"=w885:dbl, "stimulus offset"=w886:dbl, "Plant Parameters"=w883:T4)  [unwired: 4 in]
      }
      frame "Chien-Hrones-Reswick" {
        n383 = call-poly <vilib>:"PID Autotuning Design.vi"("Tuning specifications"="Tuning specifications 2", "Type of Controller"=w890, "dt (s)"=w893, "Response signal"=w896, "Stimulus signal"=w897) -> ("PID gains"=w891:T2, "response offset"=w894:dbl, "stimulus offset"=w895:dbl, "Plant Parameters"=w892:T4)  [unwired: 3 in]
      }
      frame "Internal Model Control" {
        n384 = call-poly <vilib>:"PID Autotuning Design.vi"("Desired Time Constant (tau_c)"="Multiplicative factor 2", "Type of Controller"=w899, "dt (s)"=w902, "Response signal"=w905, "Stimulus signal"=w906) -> ("PID gains"=w900:T2, "response offset"=w903:dbl, "stimulus offset"=w904:dbl, "Plant Parameters"=w901:T4)  [unwired: 3 in]
      }
    }
    "Stimulus operating point 2" <- w858
    "Response operating point 2" <- w857
    "Identified Plant Parameters 2" <- w856
    n385 = Unbundle(w861) -> ("proportional gain (Kc)"=w864:dbl)  [unwired: 2 out]
    n386 = Equal?(x=w864, y=inf) -> (x = y?=w863:bool)
    n387 = feedback #17() -> (w862:T2)  [unwired: 1 in]
    n388 = Select(t=w862, s=w863, f=w861) -> (s? t:f=w860:T2)
    "Tuned PID gains 2" <- w860
    n389 = feedback-in #17(w860) -> ()
    n390 = case shown="True" "Accept gain 2" {
      tunnel: w860 -> [_ w907]
      frame False {
      }
      frame True {
        n391 = local write "PID Gains 2"(w907) -> ()
      }
    }
    n392 = local read "Stop 2"() -> (w869:bool)
  }
  n393 = while {
    tunnel: w87 -> [_]
    tunnel: w83 -> [w911]
    stop <- w921 stop-if-true
    # "If dT and deadtime have similar values, the identification could evaluate deadtime as zero and this generates proportional gain equal to Inf. This code avoid gain changes in this situations."
    # "Autotuning Loop"
    n394 = local read "Control Output"() -> (w923:dbl[])
    n395 = local read "Measurement"() -> (w922:dbl[])
    n396 = case shown="\"Chien-Hrones-Reswick\"" "Control" {
      tunnel: w923 -> [w932 w940 w949 w958]
      tunnel: w922 -> [w931 w939 w948 w957]
      tunnel: [w930 w938 w947 w956] -> w910
      tunnel: [w929 w937 w946 w955] -> w909
      tunnel: w911 -> [w928 w936 w945 w954]
      tunnel: [w927 w935 w944 w953] -> w908
      tunnel: [w926 w934 w943 w952] -> w913
      tunnel: "Type of controller" -> [w925 w933 w942 w951]
      frame "Ziegler-Nichols", Default {
        n397 = call-poly <vilib>:"PID Autotuning Design.vi"("Ziegler-Nichols Speed"="Ziegler-Nichols speed", "Type of Controller"=w925, "dt (s)"=w928, "Response signal"=w931, "Stimulus signal"=w932) -> ("PID gains"=w926:T2, "response operating point"=w929:dbl, "stimulus operating point"=w930:dbl, "Plant Parameters"=w927:T4)  [unwired: 3 in]
      }
      frame "Cohen-Coon" {
        n398 = call-poly <vilib>:"PID Autotuning Design.vi"("Type of Controller"=w933, "dt (s)"=w936, "Response signal"=w939, "Stimulus signal"=w940) -> ("PID gains"=w934:T2, "response offset"=w937:dbl, "stimulus offset"=w938:dbl, "Plant Parameters"=w935:T4)  [unwired: 4 in]
      }
      frame "Chien-Hrones-Reswick" {
        n399 = call-poly <vilib>:"PID Autotuning Design.vi"("Tuning specifications"="Tuning specifications", "Type of Controller"=w942, "dt (s)"=w945, "Response signal"=w948, "Stimulus signal"=w949) -> ("PID gains"=w943:T2, "response offset"=w946:dbl, "stimulus offset"=w947:dbl, "Plant Parameters"=w944:T4)  [unwired: 3 in]
      }
      frame "Internal Model Control" {
        n400 = call-poly <vilib>:"PID Autotuning Design.vi"("Desired Time Constant (tau_c)"="Multiplicative factor", "Type of Controller"=w951, "dt (s)"=w954, "Response signal"=w957, "Stimulus signal"=w958) -> ("PID gains"=w952:T2, "response offset"=w955:dbl, "stimulus offset"=w956:dbl, "Plant Parameters"=w953:T4)  [unwired: 3 in]
      }
    }
    "Stimulus operating point" <- w910
    "Response operating point" <- w909
    "Identified Plant Parameters" <- w908
    n401 = Unbundle(w913) -> ("proportional gain (Kc)"=w916:dbl)  [unwired: 2 out]
    n402 = Equal?(x=w916, y=inf) -> (x = y?=w915:bool)
    n403 = feedback #18() -> (w914:T2)  [unwired: 1 in]
    n404 = Select(t=w914, s=w915, f=w913) -> (s? t:f=w912:T2)
    "Tuned PID gains" <- w912
    n405 = feedback-in #18(w912) -> ()
    n406 = case shown="True" "Accept gain" {
      tunnel: w912 -> [_ w959]
      frame False {
      }
      frame True {
        n407 = local write "PID Gains"(w959) -> ()
      }
    }
    n408 = local read "Stop"() -> (w921:bool)
  }
  n409 = while {
    shift-right: [w967] -> w79
    shift-left: w78 -> [w963]
    tunnel: w77 -> [w962]
    tunnel: [w964] -> w80
    stop <- w965 stop-if-true
    # "Serial Read Loop"
    n410 = case shown="True" TRUE {
      tunnel: [w979 w983] -> w967
      tunnel: w963 -> [w981 w983]
      tunnel: [w978 w982] -> w964
      tunnel: w962 -> [w980 w982]
      frame True {
        n411 = VISA Read(VISA resource name=w981, byte count=u32 1000, error in (no error)=w980) -> (VISA resource name out=w979:refnum<visa-resource-name>, read buffer=w976:string, error out=w978:errorcluster)  [unwired: 1 out]
        n412 = Decimal String To Number(string=w976) -> (number=w974:i32)  [unwired: 2 in, 1 out]
        "Sensor Raw Value" <- w974
        n413 = call <vilib>:"Median PtByPt.vi"("sample length"=20, "x"=w974) -> ("median"=w972:dbl)  [unwired: 2 in, 1 out]
        n414 = To Double Precision Float(number=w972) -> (double precision float=w968:dbl)
        n415 = Multiply(x=w968, y=0.0292) -> (x*y=w971:dbl)
        "Force in Kilograms 2" <- w971
        n416 = Multiply(x=w971, y=9.81) -> (x*y=→"Force in Newtons 2":dbl)
      }
      frame False {
      }
    }
    n417 = Wait (ms)(milliseconds to wait=u32 5) -> ()  [unwired: 1 out]
    n418 = Or(x=w964, y=FALSE) -> (x .or. y?=w965:bool)
  }
  n419 = while {
    shift-right: [w991] -> w47
    shift-left: w73 -> [w987]
    tunnel: w72 -> [w986]
    tunnel: [w988] -> w74
    stop <- w989 stop-if-true
    # "Serial Read Loop"
    n420 = case shown="True" TRUE {
      tunnel: [w1003 w1007] -> w991
      tunnel: w987 -> [w1005 w1007]
      tunnel: [w1002 w1006] -> w988
      tunnel: w986 -> [w1004 w1006]
      frame True {
        n421 = VISA Read(VISA resource name=w1005, byte count=u32 1000, error in (no error)=w1004) -> (VISA resource name out=w1003:refnum<visa-resource-name>, read buffer=w1000:string, error out=w1002:errorcluster)  [unwired: 1 out]
        n422 = Decimal String To Number(string=w1000) -> (number=w996:i32)  [unwired: 2 in, 1 out]
        "Sensor Raw Value 2" <- w996
        n423 = call <vilib>:"Median PtByPt.vi"("sample length"=20, "x"=w996) -> ("median"=w997:dbl)  [unwired: 2 in, 1 out]
        n424 = To Double Precision Float(number=w997) -> (double precision float=w993:dbl)
        n425 = Multiply(x=w993, y=0.0238) -> (x*y=w992:dbl)
        "Force in Kilograms" <- w992
        n426 = Multiply(x=w992, y=9.81) -> (x*y=→"Force in Newtons":dbl)
      }
      frame False {
      }
    }
    n427 = Or(x=w988, y=FALSE) -> (x .or. y?=w989:bool)
    n428 = Wait (ms)(milliseconds to wait=u32 5) -> ()  [unwired: 1 out]
  }
  n429 = while {
    stop <- FALSE stop-if-true
    # "TRACKER 4"
    # "TRACKER 3"
    # "TRACKER 2"
    # "TRACKER 1"
    n430 = Index Array(array="XYZAER", index #1=0 ("index"), index #2=1 ("index"), index #3=2 ("index"), index #4=3 ("index")) -> (element #1=w1032:T8, element #2=w1031:T8, element #3=w1030:T8, element #4=w1029:T8)
    n431 = Unbundle By Name(w1032) -> ("x"=w1019:sgl, "y"=w1018:sgl)  [unwired: 1 out]
    n432 = Unbundle By Name(w1031) -> ("x"=w1016:sgl, "y"=w1015:sgl)  [unwired: 1 out]
    n433 = Multiply(x=w1018, y=sgl -1.0) -> (x*y=w1017:sgl)
    n434 = Multiply(x=w1015, y=-1.0) -> (x*y=w1014:dbl)
    n435 = Bundle(w1014, "x"=w1016) -> (w1027:cluster{dbl, "x":sgl})  [unwired: 1 in]
    n436 = Bundle(w1017, "x"=w1019) -> (w1028:cluster{sgl, "x":sgl})  [unwired: 1 in]
    n437 = Unbundle By Name(w1030) -> ("x"=w1013:sgl, "y"=w1012:sgl)  [unwired: 1 out]
    n438 = Unbundle By Name(w1029) -> ("x"=w1010:sgl, "y"=w1009:sgl)  [unwired: 1 out]
    n439 = Multiply(x=w1012, y=-1.0) -> (x*y=w1011:dbl)
    n440 = Multiply(x=w1009, y=-1.0) -> (x*y=w1008:dbl)
    n441 = Bundle(w1011, "x"=w1013) -> (w1026:cluster{dbl, "x":sgl})  [unwired: 1 in]
    n442 = Bundle(w1008, "x"=w1010) -> (w1025:cluster{dbl, "x":sgl})  [unwired: 1 in]
    n443 = Build Array(w1028, w1027, w1026, w1025) -> (→"Position Sensor Data":cluster{dbl, "x":sgl}[])
  }
  n444 = call <instrlib>:"PDI util stationcount.vi"("error in (no error)"=w53, "pDev"=w54) -> ("error out"=w52:errorcluster, "dup pDev"=w51:u32, "MaxCount"=w49:i32)  [unwired: 7 out]
  n445 = call <instrlib>:"PDI config setbuffer.vi"("error in (no error)"=w52, "Max sensors"=w49, "FrameCount"=w50, "pDev"=w51) -> ("error out"=w61:errorcluster, "dup pDev"=w62:u32)  [unwired: 6 out]
  n446 = flat-sequence {
    tunnel: w67 -> [_]
    tunnel: [w1039] -> w63
    frame #0 {
      # "Get Start Time"
      n447 = Get Date/Time In Seconds() -> (seconds since 1Jan1904=w1040:timestamp)
      n448 = Format Date/Time String(seconds (now)=w1040) -> (date/time string=w1041:string)  [unwired: 2 out]
      n449 = local write "Start Time Text"(w1041) -> ()
      n450 = To Double Precision Float(number=w1040) -> (double precision float=w1039:dbl)
    }
  }
  n451 = call <instrlib>:"PDI action startcont.vi"("error in (no error)"=w61, "pDev"=w62) -> ("error out"=w68:errorcluster, "Running"=w60:bool, "dup pDev"=w67:u32)  [unwired: 7 out]
  n452 = control-ref of="HostFrameCount"() -> (w58:refnum<vi>)
  n453 = local write "Running"(w60) -> ()
  n454 = control-ref of="stop"() -> (w66:refnum<vi>)
  n455 = control-ref of="XYZAER"() -> (w57:refnum<vi>)
  n456 = control-ref of="PnoData"() -> (w48:refnum<vi>)
  n457 = call <instrlib>:"PDI data xyzaer loop.vi"("Data Ready Refnum"=w48, "FrameCount Ctl Ref"=w58, "error in (no error)"=w68, "xyzaer array\nRefnum"=w57, "Stop Ctl Ref"=w66, "pDev"=w67) -> ("error out"=w55:errorcluster, "Loop Iter"=w59:i32, "dup pDev"=w56:u32)  [unwired: 3 out]
  n458 = local write "Loop Iter"(w59) -> ()
  n459 = call <instrlib>:"PDI action stopcont.vi"("error in (no error)"=w55, "pDev"=w56) -> ("error out"=w64:errorcluster, "Running"=w69:bool, "dup pDev"=w70:u32)  [unwired: 7 out]
  n460 = local write "Running"(w69) -> ()
  n461 = case shown="No Error" w55 {
    tunnel: w63 -> [w1042 _]
    frame No Error {
      # "Success up to here"
      n462 = call "Elapsed Time"("Set Start Time (s)"=w1042) -> ("Present Text"=w1044:string, "Elapsed Time Text"=w1043:string)  [unwired: 4 in, 13 out]
      n463 = local write "Stop Time Text"(w1044) -> ()
      n464 = local write "Elapsed Time Text"(w1043) -> ()
    }
    frame Error {
      # "Error somewhere;\nStop Time is irrelevant"
    }
  }
  n465 = call <instrlib>:"PDI close.vi"("error in (no error)"=w64, "pDev"=w70) -> ("error out"=→"error out":errorcluster, "connected"=w65:bool)  [unwired: 8 out]
  n466 = local write "Connected"(w65) -> ()
  n467 = VISA Close(VISA resource name=w79, error in (no error)=w80) -> (error out=w81:errorcluster)
  n468 = call <vilib>:"Simple Error Handler.vi"("error in (no error)"=w81) -> ()  [unwired: 1 in, 8 out]
  n469 = VISA Close(VISA resource name=w47, error in (no error)=w74) -> (error out=w75:errorcluster)
  n470 = call <vilib>:"Simple Error Handler.vi"("error in (no error)"=w75) -> ()  [unwired: 1 in, 8 out]
  n471 = Compound Arithmetic op=OR(FALSE, w46) -> (w45:bool)
  n472 = case shown="True" w45 {
    frame False {
    }
    frame True {
      n473 = call <vilib>:"Beep.vi"("use system alert? (T)"=FALSE, "duration (msec)"=u32 2000, "frequency (Hz)"=u32 15000) -> ()  [unwired: 9 in]
    }
  }
  n474 = while {
    shift-left: 0.0 ("Plant Output") -> [w1112]
    shift-right: [w1107] -> _
    tunnel: w6 -> [_]
    shift-right: [w1093] -> _
    shift-left: 0.01 -> [w1091]
    shift-right: [w1065] -> _
    shift-left: TRUE -> [w1090]
    shift-right: [w1067] -> _
    shift-left: w3 -> [w1089]
    shift-right: [w1092] -> _
    shift-left: w3 -> [w1088]
    tunnel: [w1062] -> w2
    tunnel: w1 -> [w1048]
    stop <- "Stop 8" stop-if-true
    w1053 = 1 items=["one channel for each line", "one channel for all lines"] ("line grouping")
    w1062 = 0.05 ("Sampling Time dt (s)")
    w1071 = 1 items=["one channel for each line", "one channel for all lines"] ("line grouping")
    w1079 = 0.5 ("x")
    w1106 = T7 {"static gain"=2.5, "lag (s)"=2.5, "deadtime (s)"=0.01, "load"=0.0, "deadband"=0.0, "sensor noise"=0.0, "initial PV"=30.0, "plant noise"=0.0}  # Process parameters
    w1108 = FALSE  # Integrator ?
    # "C."
    # "Inlet 11"
    # "Exhaust 2"
    # "B."
    # "A."
    # "A.Output to PWM Logic \nB. Simulated Plant\nC. Draw Chart"
    # "Main PID Loop Control"
    n475 = Multiply(x=w1062, y=1000.0) -> (x*y=w1105:dbl)
    n476 = Not(x="Autotune 8") -> (.not. x?=w1109:bool)
    n477 = feedback #19() -> (w1114:bool)  [unwired: 1 in]
    n478 = feedback-in #19("Autotune 8") -> ()
    n479 = Wait Until Next ms Multiple(millisecond multiple=w1105) -> ()  [unwired: 1 out]
    n480 = Exclusive Or(1:w1114, 2:"Autotune 8") -> (0:w1113:bool)
    n481 = feedback #20() -> (w1111:dbl)  [unwired: 1 in]
    n482 = Multiply(x=w1048, y=-1000.0) -> (x*y=w1095:dynamicdata)
    n483 = call <vilib>:"Median PtByPt.vi"("sample length"="Median sample length 17", "x"=w1095) -> ("median"=w1094:dbl)  [unwired: 2 in, 1 out]
    n484 = Square(x=w1094) -> (x^2=w1102:dbl)
    n485 = Multiply(x=w1094, y=-39.646) -> (x*y=w1098:dbl)
    n486 = Multiply(x=w1102, y=0.2324) -> (x*y=w1099:dbl)
    n487 = Add(x=w1098, y=w1099) -> (x+y=w1097:dbl)
    n488 = Add(x=1678.0, y=w1097) -> (x+y=w1060:dbl)
    n489 = case shown="False" "Autotune 8" {
      tunnel: w1062 -> [w1129 _]
      tunnel: [w1118 w1134] -> w1067
      tunnel: w1112 -> [_ w1133]
      tunnel: "PID Gains 8" -> [w1128 _]
      tunnel: "Reinitialize 8" -> [w1125 _]
      tunnel: w1113 -> [w1127 w1132]
      tunnel: w1111 -> [_ w1136]
      tunnel: w1060 -> [w1121 _]
      tunnel: "Set Point 8" -> [w1120 _]
      frame False {
        # "This code is to have 'bumpless' transfer from autotuning"
        n490 = Not(x=w1127) -> (.not. x?=w1124:bool)
        n491 = And(x="Automatic 8", y=w1124) -> (x .and. y?=w1126:bool)
        n492 = call-poly <vilib>:"PID Advanced.vi"("setpoint"=w1120, "auto? (T)"=w1126, "manual control"="MV: 8", "process variable"=w1121, "alpha"=10.0, "PID gains"=w1128, "dt (s)"=w1129, "reinitialize? (F)"=w1125) -> ("output"=w1118:dbl)  [unwired: 6 in, 1 out]
      }
      frame True {
        w1139 = 10000 ("sample length")
        # "Buffering data for parameters estimation"
        n493 = call <vilib>:"Data Queue PtByPt.vi"("initial queue element"=w1133, "initialize"=w1132, "sample length"=w1139, "input data point"=w1133) -> ("Current Queue"=→"Control Output 8":dbl[])  [unwired: 3 in, 4 out]
        n494 = Select(t=0.0, s=w1132, f="Excitation 8") -> (s? t:f=w1137:dbl)
        n495 = Add(x=w1136, y=w1137) -> (x+y=w1134:dbl)
        n496 = call <vilib>:"Data Queue PtByPt.vi"("initial queue element"=w1134, "initialize"=w1132, "sample length"=w1139, "input data point"=w1134) -> ("Current Queue"=→"Measurement 8":dbl[])  [unwired: 3 in, 4 out]
      }
    }
    n497 = feedback-in #20(w1067, w1109) -> ()
    n498 = Greater?(x=w1060, y="M-2") -> ()  [unwired: 1 out]
    n499 = Add(x=w1091, y=w1079) -> (x+y=w1080:dbl)
    n500 = Subtract(x=w1091, y=w1079) -> (x-y=w1078:dbl)
    n501 = Equal?(x=w1089, y=w1067) -> (x = y?=w1086:bool)
    n502 = Greater?(x=w1067, y=w1089) -> (0:w1085:bool)
    n503 = Select(t=w1090, s=w1086, f=w1085) -> (s? t:f=w1065:bool)
    "PWM Output 8" <- w1065
    n504 = call "Plant System.vi"("Integrator ?"=w1108, "Plant Input"=w1067, "dt (s)"=w1062, "process parameters"=w1106) -> ("Plant Output"=w1107:dbl)  [unwired: 11 in]
    n505 = Increment(x="Set Point 8") -> (x+1=w1084:dbl)
    n506 = Decrement(x="Set Point 8") -> (x-1=w1083:dbl)
    n507 = Select(t=w1080, s=w1065, f=w1078) -> (s? t:f=w1093:dbl)
    n508 = Select(t=w1084, s=w1065, f=w1083) -> (s? t:f=w1082:dbl)
    n509 = Not(x=w1065) -> (.not. x?=w1064:bool)
    n510 = call-poly <vilib>:"DAQmx Create Virtual Channel.vi"("lines"=tag "cDAQ1Mod1/port0/line6", "line grouping"=w1071) -> ("task out"=w1073:refnum<k21>, "error out"=w1072:errorcluster)  [unwired: 12 in]
    n511 = call-poly <vilib>:"DAQmx Create Virtual Channel.vi"("lines"=tag "cDAQ1Mod2/port0/line6", "line grouping"=w1053) -> ("task out"=w1055:refnum<k21>, "error out"=w1054:errorcluster)  [unwired: 12 in]
    n512 = Build Array(w1060, "Set Point 8", w1082) -> (w1081:dbl[])
    n513 = Initialize Array("INLET 2 ON/OFF 2", 1 ("dimension size")) -> (w1050:bool[])
    n514 = Initialize Array(w1064, 1 ("dimension size")) -> (w1068:bool[])
    n515 = local write "MV: 8"(w1067) -> ()
    n516 = Add(x=w1088, y=w1091) -> (x+y=w1092:dbl)
    n517 = Build Array(w1081) -> (→"Real time Data 8":dbl[][])
    n518 = call-poly <vilib>:"DAQmx Write.vi"("task/channels in"=w1073, "auto start"=TRUE, "data"=w1068, "error in"=w1072) -> ("task out"=w1075:refnum<k21>, "error out"=w1076:errorcluster)  [unwired: 9 in, 1 out]
    n519 = call-poly <vilib>:"DAQmx Write.vi"("task/channels in"=w1055, "auto start"=TRUE, "data"=w1050, "error in"=w1054) -> ("task out"=w1057:refnum<k21>, "error out"=w1058:errorcluster)  [unwired: 9 in, 1 out]
    n520 = call <vilib>:"DAQmx Clear Task.vi"("task in"=w1075, "error in"=w1076) -> ("error out"=w1070:errorcluster)  [unwired: 13 in]
    n521 = call <vilib>:"DAQmx Clear Task.vi"("task in"=w1057, "error in"=w1058) -> ("error out"=w1052:errorcluster)  [unwired: 13 in]
    n522 = call <vilib>:"Simple Error Handler.vi"("error in (no error)"=w1070) -> ()  [unwired: 4 in, 5 out]
    n523 = call <vilib>:"Simple Error Handler.vi"("error in (no error)"=w1052) -> ()  [unwired: 4 in, 5 out]
  }
  n524 = while {
    shift-left: 0.0 ("Plant Output") -> [w1204]
    shift-right: [w1199] -> _
    tunnel: w12 -> [_]
    shift-right: [w1185] -> _
    shift-left: 0.01 -> [w1183]
    shift-right: [w1157] -> _
    shift-left: TRUE -> [w1182]
    shift-right: [w1159] -> _
    shift-left: w9 -> [w1181]
    shift-right: [w1184] -> _
    shift-left: w9 -> [w1180]
    tunnel: [w1154] -> w8
    tunnel: w1 -> [w1140]
    stop <- "Stop 7" stop-if-true
    w1145 = 1 items=["one channel for each line", "one channel for all lines"] ("line grouping")
    w1154 = 0.05 ("Sampling Time dt (s)")
    w1163 = 1 items=["one channel for each line", "one channel for all lines"] ("line grouping")
    w1171 = 0.5 ("x")
    w1198 = T7 {"static gain"=2.5, "lag (s)"=2.5, "deadtime (s)"=0.01, "load"=0.0, "deadband"=0.0, "sensor noise"=0.0, "initial PV"=30.0, "plant noise"=0.0}  # Process parameters
    w1200 = FALSE  # Integrator ?
    # "C."
    # "Inlet 11"
    # "Exhaust 7"
    # "B."
    # "A."
    # "A.Output to PWM Logic \nB. Simulated Plant\nC. Draw Chart"
    # "Main PID Loop Control"
    n525 = Multiply(x=w1154, y=1000.0) -> (x*y=w1197:dbl)
    n526 = Not(x="Autotune 7") -> (.not. x?=w1201:bool)
    n527 = feedback #21() -> (w1206:bool)  [unwired: 1 in]
    n528 = feedback-in #21("Autotune 7") -> ()
    n529 = Wait Until Next ms Multiple(millisecond multiple=w1197) -> ()  [unwired: 1 out]
    n530 = Exclusive Or(1:w1206, 2:"Autotune 7") -> (0:w1205:bool)
    n531 = feedback #22() -> (w1203:dbl)  [unwired: 1 in]
    n532 = Multiply(x=w1140, y=-1000.0) -> (x*y=w1187:dynamicdata)
    n533 = call <vilib>:"Median PtByPt.vi"("sample length"="Median sample length 16", "x"=w1187) -> ("median"=w1186:dbl)  [unwired: 2 in, 1 out]
    n534 = Square(x=w1186) -> (x^2=w1194:dbl)
    n535 = Multiply(x=w1186, y=-39.646) -> (x*y=w1190:dbl)
    n536 = Multiply(x=w1194, y=0.2324) -> (x*y=w1191:dbl)
    n537 = Add(x=w1190, y=w1191) -> (x+y=w1189:dbl)
    n538 = Add(x=1678.0, y=w1189) -> (x+y=w1152:dbl)
    n539 = case shown="False" "Autotune 7" {
      tunnel: w1154 -> [w1221 _]
      tunnel: [w1210 w1226] -> w1159
      tunnel: w1204 -> [_ w1225]
      tunnel: "PID Gains 7" -> [w1220 _]
      tunnel: "Reinitialize 7" -> [w1217 _]
      tunnel: w1205 -> [w1219 w1224]
      tunnel: w1203 -> [_ w1228]
      tunnel: w1152 -> [w1213 _]
      tunnel: "Set Point 7" -> [w1212 _]
      frame False {
        # "This code is to have 'bumpless' transfer from autotuning"
        n540 = Not(x=w1219) -> (.not. x?=w1216:bool)
        n541 = And(x="Automatic 7", y=w1216) -> (x .and. y?=w1218:bool)
        n542 = call-poly <vilib>:"PID Advanced.vi"("setpoint"=w1212, "auto? (T)"=w1218, "manual control"="MV: 7", "process variable"=w1213, "alpha"=10.0, "PID gains"=w1220, "dt (s)"=w1221, "reinitialize? (F)"=w1217) -> ("output"=w1210:dbl)  [unwired: 6 in, 1 out]
      }
      frame True {
        w1231 = 10000 ("sample length")
        # "Buffering data for parameters estimation"
        n543 = call <vilib>:"Data Queue PtByPt.vi"("initial queue element"=w1225, "initialize"=w1224, "sample length"=w1231, "input data point"=w1225) -> ("Current Queue"=→"Control Output 7":dbl[])  [unwired: 3 in, 4 out]
        n544 = Select(t=0.0, s=w1224, f="Excitation 7") -> (s? t:f=w1229:dbl)
        n545 = Add(x=w1228, y=w1229) -> (x+y=w1226:dbl)
        n546 = call <vilib>:"Data Queue PtByPt.vi"("initial queue element"=w1226, "initialize"=w1224, "sample length"=w1231, "input data point"=w1226) -> ("Current Queue"=→"Measurement 7":dbl[])  [unwired: 3 in, 4 out]
      }
    }
    n547 = feedback-in #22(w1159, w1201) -> ()
    n548 = Greater?(x=w1152, y="M-7") -> ()  [unwired: 1 out]
    n549 = Add(x=w1183, y=w1171) -> (x+y=w1172:dbl)
    n550 = Subtract(x=w1183, y=w1171) -> (x-y=w1170:dbl)
    n551 = Equal?(x=w1181, y=w1159) -> (x = y?=w1178:bool)
    n552 = Greater?(x=w1159, y=w1181) -> (0:w1177:bool)
    n553 = Select(t=w1182, s=w1178, f=w1177) -> (s? t:f=w1157:bool)
    "PWM Output 7" <- w1157
    n554 = call "Plant System.vi"("Integrator ?"=w1200, "Plant Input"=w1159, "dt (s)"=w1154, "process parameters"=w1198) -> ("Plant Output"=w1199:dbl)  [unwired: 11 in]
    n555 = Increment(x="Set Point 7") -> (x+1=w1176:dbl)
    n556 = Decrement(x="Set Point 7") -> (x-1=w1175:dbl)
    n557 = Select(t=w1172, s=w1157, f=w1170) -> (s? t:f=w1185:dbl)
    n558 = Select(t=w1176, s=w1157, f=w1175) -> (s? t:f=w1174:dbl)
    n559 = Not(x=w1157) -> (.not. x?=w1156:bool)
    n560 = call-poly <vilib>:"DAQmx Create Virtual Channel.vi"("lines"=tag "cDAQ1Mod8/port0/line6", "line grouping"=w1163) -> ("task out"=w1165:refnum<k21>, "error out"=w1164:errorcluster)  [unwired: 12 in]
    n561 = call-poly <vilib>:"DAQmx Create Virtual Channel.vi"("lines"=tag "cDAQ1Mod7/port0/line5", "line grouping"=w1145) -> ("task out"=w1147:refnum<k21>, "error out"=w1146:errorcluster)  [unwired: 12 in]
    n562 = Build Array(w1152, "Set Point 7", w1174) -> (w1173:dbl[])
    n563 = Initialize Array("INLET 7 ON/OFF 2", 1 ("dimension size")) -> (w1142:bool[])
    n564 = Initialize Array(w1156, 1 ("dimension size")) -> (w1160:bool[])
    n565 = local write "MV: 7"(w1159) -> ()
    n566 = Add(x=w1180, y=w1183) -> (x+y=w1184:dbl)
    n567 = Build Array(w1173) -> (→"Real time Data 7":dbl[][])
    n568 = call-poly <vilib>:"DAQmx Write.vi"("task/channels in"=w1165, "auto start"=TRUE, "data"=w1160, "error in"=w1164) -> ("task out"=w1167:refnum<k21>, "error out"=w1168:errorcluster)  [unwired: 9 in, 1 out]
    n569 = call-poly <vilib>:"DAQmx Write.vi"("task/channels in"=w1147, "auto start"=TRUE, "data"=w1142, "error in"=w1146) -> ("task out"=w1149:refnum<k21>, "error out"=w1150:errorcluster)  [unwired: 9 in, 1 out]
    n570 = call <vilib>:"DAQmx Clear Task.vi"("task in"=w1167, "error in"=w1168) -> ("error out"=w1162:errorcluster)  [unwired: 13 in]
    n571 = call <vilib>:"DAQmx Clear Task.vi"("task in"=w1149, "error in"=w1150) -> ("error out"=w1144:errorcluster)  [unwired: 13 in]
    n572 = call <vilib>:"Simple Error Handler.vi"("error in (no error)"=w1162) -> ()  [unwired: 4 in, 5 out]
    n573 = call <vilib>:"Simple Error Handler.vi"("error in (no error)"=w1144) -> ()  [unwired: 4 in, 5 out]
  }
  n574 = local write "Stop 8"(w6) -> ()
  n575 = local write "Stop 7"(w12) -> ()
  n576 = while {
    tunnel: w6 -> [_]
    tunnel: w2 -> [w1235]
    stop <- w1245 stop-if-true
    # "If dT and deadtime have similar values, the identification could evaluate deadtime as zero and this generates proportional gain equal to Inf. This code avoid gain changes in this situations."
    # "Autotuning Loop"
    n577 = local read "Control Output 8"() -> (w1247:dbl[])
    n578 = local read "Measurement 8"() -> (w1246:dbl[])
    n579 = case shown="\"Chien-Hrones-Reswick\"" "Control 8" {
      tunnel: w1247 -> [w1256 w1264 w1273 w1282]
      tunnel: w1246 -> [w1255 w1263 w1272 w1281]
      tunnel: [w1254 w1262 w1271 w1280] -> w1234
      tunnel: [w1253 w1261 w1270 w1279] -> w1233
      tunnel: w1235 -> [w1252 w1260 w1269 w1278]
      tunnel: [w1251 w1259 w1268 w1277] -> w1232
      tunnel: [w1250 w1258 w1267 w1276] -> w1237
      tunnel: "Type of controller 8" -> [w1249 w1257 w1266 w1275]
      frame "Ziegler-Nichols", Default {
        n580 = call-poly <vilib>:"PID Autotuning Design.vi"("Ziegler-Nichols Speed"="Ziegler-Nichols speed 8", "Type of Controller"=w1249, "dt (s)"=w1252, "Response signal"=w1255, "Stimulus signal"=w1256) -> ("PID gains"=w1250:T2, "response operating point"=w1253:dbl, "stimulus operating point"=w1254:dbl, "Plant Parameters"=w1251:T4)  [unwired: 3 in]
      }
      frame "Cohen-Coon" {
        n581 = call-poly <vilib>:"PID Autotuning Design.vi"("Type of Controller"=w1257, "dt (s)"=w1260, "Response signal"=w1263, "Stimulus signal"=w1264) -> ("PID gains"=w1258:T2, "response offset"=w1261:dbl, "stimulus offset"=w1262:dbl, "Plant Parameters"=w1259:T4)  [unwired: 4 in]
      }
      frame "Chien-Hrones-Reswick" {
        n582 = call-poly <vilib>:"PID Autotuning Design.vi"("Tuning specifications"="Tuning specifications 8", "Type of Controller"=w1266, "dt (s)"=w1269, "Response signal"=w1272, "Stimulus signal"=w1273) -> ("PID gains"=w1267:T2, "response offset"=w1270:dbl, "stimulus offset"=w1271:dbl, "Plant Parameters"=w1268:T4)  [unwired: 3 in]
      }
      frame "Internal Model Control" {
        n583 = call-poly <vilib>:"PID Autotuning Design.vi"("Desired Time Constant (tau_c)"="Multiplicative factor 8", "Type of Controller"=w1275, "dt (s)"=w1278, "Response signal"=w1281, "Stimulus signal"=w1282) -> ("PID gains"=w1276:T2, "response offset"=w1279:dbl, "stimulus offset"=w1280:dbl, "Plant Parameters"=w1277:T4)  [unwired: 3 in]
      }
    }
    "Stimulus operating point 8" <- w1234
    "Response operating point 8" <- w1233
    "Identified Plant Parameters 8" <- w1232
    n584 = Unbundle(w1237) -> ("proportional gain (Kc)"=w1240:dbl)  [unwired: 2 out]
    n585 = Equal?(x=w1240, y=inf) -> (x = y?=w1239:bool)
    n586 = feedback #23() -> (w1238:T2)  [unwired: 1 in]
    n587 = Select(t=w1238, s=w1239, f=w1237) -> (s? t:f=w1236:T2)
    "Tuned PID gains 8" <- w1236
    n588 = feedback-in #23(w1236) -> ()
    n589 = case shown="True" "Accept gain 8" {
      tunnel: w1236 -> [_ w1283]
      frame False {
      }
      frame True {
        n590 = local write "PID Gains 8"(w1283) -> ()
      }
    }
    n591 = local read "Stop 8"() -> (w1245:bool)
  }
  n592 = while {
    tunnel: w12 -> [_]
    tunnel: w8 -> [w1287]
    stop <- w1297 stop-if-true
    # "If dT and deadtime have similar values, the identification could evaluate deadtime as zero and this generates proportional gain equal to Inf. This code avoid gain changes in this situations."
    # "Autotuning Loop"
    n593 = local read "Control Output 7"() -> (w1299:dbl[])
    n594 = local read "Measurement 7"() -> (w1298:dbl[])
    n595 = case shown="\"Chien-Hrones-Reswick\"" "Control 7" {
      tunnel: w1299 -> [w1308 w1316 w1325 w1334]
      tunnel: w1298 -> [w1307 w1315 w1324 w1333]
      tunnel: [w1306 w1314 w1323 w1332] -> w1286
      tunnel: [w1305 w1313 w1322 w1331] -> w1285
      tunnel: w1287 -> [w1304 w1312 w1321 w1330]
      tunnel: [w1303 w1311 w1320 w1329] -> w1284
      tunnel: [w1302 w1310 w1319 w1328] -> w1289
      tunnel: "Type of controller 7" -> [w1301 w1309 w1318 w1327]
      frame "Ziegler-Nichols", Default {
        n596 = call-poly <vilib>:"PID Autotuning Design.vi"("Ziegler-Nichols Speed"="Ziegler-Nichols speed 7", "Type of Controller"=w1301, "dt (s)"=w1304, "Response signal"=w1307, "Stimulus signal"=w1308) -> ("PID gains"=w1302:T2, "response operating point"=w1305:dbl, "stimulus operating point"=w1306:dbl, "Plant Parameters"=w1303:T4)  [unwired: 3 in]
      }
      frame "Cohen-Coon" {
        n597 = call-poly <vilib>:"PID Autotuning Design.vi"("Type of Controller"=w1309, "dt (s)"=w1312, "Response signal"=w1315, "Stimulus signal"=w1316) -> ("PID gains"=w1310:T2, "response offset"=w1313:dbl, "stimulus offset"=w1314:dbl, "Plant Parameters"=w1311:T4)  [unwired: 4 in]
      }
      frame "Chien-Hrones-Reswick" {
        n598 = call-poly <vilib>:"PID Autotuning Design.vi"("Tuning specifications"="Tuning specifications 7", "Type of Controller"=w1318, "dt (s)"=w1321, "Response signal"=w1324, "Stimulus signal"=w1325) -> ("PID gains"=w1319:T2, "response offset"=w1322:dbl, "stimulus offset"=w1323:dbl, "Plant Parameters"=w1320:T4)  [unwired: 3 in]
      }
      frame "Internal Model Control" {
        n599 = call-poly <vilib>:"PID Autotuning Design.vi"("Desired Time Constant (tau_c)"="Multiplicative factor 7", "Type of Controller"=w1327, "dt (s)"=w1330, "Response signal"=w1333, "Stimulus signal"=w1334) -> ("PID gains"=w1328:T2, "response offset"=w1331:dbl, "stimulus offset"=w1332:dbl, "Plant Parameters"=w1329:T4)  [unwired: 3 in]
      }
    }
    "Stimulus operating point 7" <- w1286
    "Response operating point 7" <- w1285
    "Identified Plant Parameters 7" <- w1284
    n600 = Unbundle(w1289) -> ("proportional gain (Kc)"=w1292:dbl)  [unwired: 2 out]
    n601 = Equal?(x=w1292, y=inf) -> (x = y?=w1291:bool)
    n602 = feedback #24() -> (w1290:T2)  [unwired: 1 in]
    n603 = Select(t=w1290, s=w1291, f=w1289) -> (s? t:f=w1288:T2)
    "Tuned PID gains 7" <- w1288
    n604 = feedback-in #24(w1288) -> ()
    n605 = case shown="True" "Accept gain 7" {
      tunnel: w1288 -> [_ w1335]
      frame False {
      }
      frame True {
        n606 = local write "PID Gains 7"(w1335) -> ()
      }
    }
    n607 = local read "Stop 7"() -> (w1297:bool)
  }
